vi "MAIN.vi"() -> ()   [LabVIEW 2015]
doc: "Use this template to create an application that executes repeatedly until you click the Stop button. This template polls the state of the Stop button and does not use events. Use the Top-Level Application template (not available in the Base package) to create a single-loop application with event handling."
uses:
  Lib_Bled112 toolkit/type_def/connection_status_bundle.ctl
  Lib_Bled112 toolkit/type_def/address_type.ctl
  Lib_Bled112 toolkit/type_def/message_type.ctl
  Lib_Bled112 toolkit/type_def/message_class.ctl
  <vilib>/Utility/miscctls.llb/LVPointTypeDef.ctl
  SUB_Load and Save Controls.llb/RWC_Actions.ctl
  <vilib>/Utility/miscctls.llb/LVRowAndColumnTypeDef.ctl
  <vilib>/event_ctls.llb/eventvkey.ctl
  <vilib>/Utility/sysdir.llb/System Directory Type.ctl
  <vilib>/Utility/NIReport.llb/image depth.ctl
  <vilib>/Analysis/baseanly.llb/Mean (DBL).vi
  Global 1.vi
  <vilib>/Utility/config.llb/Read Key (String).vi
  <vilib>/Utility/config.llb/Read Key (I32).vi
  Lib_Bled112 toolkit/ble_functions/ble_write_by_handle_uint8array.vi
  <vilib>/addons/_office/excel.llb/Excel Easy Table (str).vi
  <vilib>/Utility/config.llb/Write Key (String).vi
  <vilib>/Utility/config.llb/Write Key (U32).vi
  <vilib>/Utility/NIReport.llb/NI_report.lvclass
  <vilib>/Utility/config.llb/NI_LVConfig.lvlib
  <vilib>/Analysis/NI_AALBase.lvlib
  <vilib>/addons/_office/NI_ReportGenerationToolkit.lvlib
  <vilib>/Utility/NIReport.llb/NI_ReportGenerationCore.lvlib
  <vilib>/Utility/NIReport.llb/Excel/NI_Excel.lvclass
  <vilib>/Analysis/NI_AALPro.lvlib
panel:
  out "ms timer 3":u32=25058615
  in  "Interval(ms)":u16
  out "ms timer 2":u32=25058615
  out "Rx-ROM":bool=TRUE
  out "BLE Packet (mon)":u8[](array[numeric])
  out "Timer-ble log":u32
  out "log data1":bool=TRUE
  out "log ble buf":string
  out "Packet Detect":bool=TRUE
  out "Disconnected":bool=TRUE
  out "Rx OK":bool=TRUE
  out "Rx buf 1":string
  out "Rx Cnt":i32=3775
  out "Rx Packet Structure":T1={"Message Type (Response)"=128, "Payload length"=0, "Command Class (System)"=1, "Message ID"=0, "Connection handle"=0, "Attribute handle"=0, "Attribute type"=1, "Attribute value (data)"=[]} {"Attribute type" format="%02x" items=["read", "notify", "indicate", "read_by_type", "read_blob", "indicate_rsp_req"]; "Attribute value (data)" format="%02x"; "Attribute handle" format="%04x"; "Connection handle" format="%02x"; "Message ID" format="%02x"; "Message Type (Response)" format="%02x" items=["Command / Response"=0, "Event"=128]; "Command Class (System)" format="%02x" items=["System", "Persistent Store", "Attribute database", "Connection", "Attribute client", "Security Manager", "Generic Access Profile", "Hardware"]}
  out "Device Name":string
  out "Connection Status":T4={"MAC Address"="D9:2F:10:92:34:F2", "cnx handle"=0, "cnx flags"=5, "Address Type"=1, "Connection Interval (ms)"=15, "Timeout(ms)"=1000, "Latency"=0, "bonding handle"=255} {"Address Type" items=["Public", "Random"]}
  in  "Log no":string="1" caption="No."
  out "FTS OP status":T6="시험 시작"
  out "Test profile":string[][](array[string])=[["Init(1)-35lb", "35", "5000"], ["Init(2)-70lb", "70", "5000"], ["Load(1)-0lb", "0", "3000"], ["Load(2)-5lb", "5", "3000"], ["Load(3)-10lb", "10", "3000"], ["Load(4)-20lb", "20", "3000"], ["Load(5)-30lb", "30", "3000"], ["Load(6)-40lb", "40", "3000"]]
  out "log refnum":refnum<file> caption="참조 번호 복제"
  out "ms timer":u32=25058615
  out "Logging No.":u32
  in  "Data Logging":bool caption="Data Logging (Desktop folder)"
  out "RxD":string
  out "Graph timer 2":u32=25058662
  out "창크게":bool
  out "Comm err cnt 1":i32
  out "Graph timer 1":u32=25058662
  in  "Setting load":bool=TRUE
  out "ACT-Comm":bool
  in  "Comm con 1":bool
  in  "Port close 1":bool
  in  "Port open 1":bool
  in  "탭-Top":T7(tab)
  out "CDC Offet":T8 caption="CDC Offset data" {"Right Wing-C, C6/C0" format="%#.9f"; "Right Wing-B, C5/C0" format="%#.9f"; "Right Wing-A, C4/C0" format="%#.9f"; "Left Wing-C, C3/C0" format="%#.9f"; "Left Wing-B, C2/C0" format="%#.9f"; "Left Wing-A, C1/C0" format="%#.9f"}
  in  "Export graph 1":bool
  in  "Clear graph 1":bool
  out "CDC(PCAP02) Graph":waveform(dbl)[](graph)=[{"t0"=timestamp(3554680480.5032296 s since 1904-01-01), "dt"=0.10200000000000001, "Y"=[0.9929709434509277]}, {"t0"=timestamp(3554680480.5032296 s since 1904-01-01), "dt"=0.10200000000000001, "Y"=[0.9975447654724121]}, {"t0"=timestamp(3554680480.5032296 s since 1904-01-01), "dt"=0.10200000000000001, "Y"=[0.9987750053405762]}, {"t0"=timestamp(3554680480.5032296 s since 1904-01-01), "dt"=0.10200000000000001, "Y"=[1.0097055435180664]}, {"t0"=timestamp(3554680480.5032296 s since 1904-01-01), "dt"=0.10200000000000001, "Y"=[1.0132465362548828]}, {"t0"=timestamp(3554680480.5032296 s since 1904-01-01), "dt"=0.10200000000000001, "Y"=[1.0090084075927734]}]
  out "CDC data":T8 caption="CDC Monitoring data" {"Right Wing-C, C6/C0" format="%#.9f"; "Right Wing-B, C5/C0" format="%#.9f"; "Right Wing-A, C4/C0" format="%#.9f"; "Left Wing-C, C3/C0" format="%#.9f"; "Left Wing-B, C2/C0" format="%#.9f"; "Left Wing-A, C1/C0" format="%#.9f"}
  in  "Offset 1":bool
  out "IMU Offet":T9 caption="IMU Offset data" {"Accelerometer Z" format="%#.9f"; "Accelerometer Y" format="%#.9f"; "Accelerometer X" format="%#.9f"; "Gyroscope Z" format="%#.9f"; "Gyroscope Y" format="%#.9f"; "Gyroscope X" format="%#.9f"}
  out "IMU Graph":waveform(dbl)[](graph)=[{"t0"=timestamp(3554680480.5032296 s since 1904-01-01), "dt"=0.10200000000000001, "Y"=[3.465625]}, {"t0"=timestamp(3554680480.5032296 s since 1904-01-01), "dt"=0.10200000000000001, "Y"=[-2.45625]}, {"t0"=timestamp(3554680480.5032296 s since 1904-01-01), "dt"=0.10200000000000001, "Y"=[-1.45875]}, {"t0"=timestamp(3554680480.5032296 s since 1904-01-01), "dt"=0.10200000000000001, "Y"=[-0.014274]}, {"t0"=timestamp(3554680480.5032296 s since 1904-01-01), "dt"=0.10200000000000001, "Y"=[0.000305]}, {"t0"=timestamp(3554680480.5032296 s since 1904-01-01), "dt"=0.10200000000000001, "Y"=[1.025959]}]
  in  "Clear graph 2":bool
  in  "Export graph2":bool
  out "IMU data":T9 caption="IMU Monitoring data" {"Accelerometer Z" format="%#.9f"; "Accelerometer Y" format="%#.9f"; "Accelerometer X" format="%#.9f"; "Gyroscope Z" format="%#.9f"; "Gyroscope Y" format="%#.9f"; "Gyroscope X" format="%#.9f"}
  in  "Offset 2":bool
  out "Full ROM data":bool
  in  "Flash Map":enum32{"Data Map", "Raw Data"}(tab)
  out "Rx ROM-log":string
  out "ROM Data":T10(array[cluster]) {"Index" format="%02x"; "ROM Data" format="%02x"}
  out "Bat(raw)":u16 format="%04x"
  in  "Load(lb)":dbl=10.0 min=0.0 max=150.0 step=0.1
  in  "Test name":string="Noname"
  out "Load vs Ratio Graph":cluster{dbl[], dbl[]}[](graph)
  in  "Mark10 Gauge (lb)":dbl format="%.2f"
  out "Test Status":string
  out "Test Data table":string[][](table)=[["-", "-", "-", "-", "-", "-", "-", "-", "-", "-"], ["-", "-", "-", "-", "-", "-", "-", "-", "-", "-"], ["-", "-", "-", "-", "-", "-", "-", "-", "-", "-"], ["-", "-", "-", "-", "-", "-", "-", "-", "-", "-"], ["-", "-", "-", "-", "-", "-", "-", "-", "-", "-"], ["-", "-", "-", "-", "-", "-", "-", "-", "-", "-"], ["-", "-", "-", "-", "-", "-", "-", "-", "-", "-"], ["-", "-", "-", "-", "-", "-", "-", "-", "-", "-"], ["-", "-", "-", "-", "-", "-", "-", "-", "-", "-"]]
  in  "Test Start":bool
  in  "Port-FTS":refnum<visa-resource-name>="COM5" caption="FTS \nCOM port"
  in  "FTS Testing":bool
  out "FTS comm.":bool
  in  "Force Set":bool
  out "Rx-mon":bool=TRUE
  out "Comm con status 1":bool caption="Status"
  out "*Board ID1":string="None...." caption="S/N"
  in  "Port-set 1":refnum<visa-resource-name>="COM4" caption="COM port"
  out "Port-act 1":refnum<visa-resource-name>="COM4"
  in  "stop":bool=TRUE
  out "Data trx(led)":bool
  in  "Setting load(led)":bool
  out "status string":string="Ready (available after the communication connection)"
  # "GEN4 2nd PP - GUI Program"
  # "Ver. 161109A"
  # "Comm. Connection"
  # "115200bps"
  # "Gyroscope X"
  # "Gyroscope Y"
  # "Gyro. (dps)"
  # "Gyroscope Z"
  # "Accelerometer X"
  # "Accelerometer Y"
  # "Acc. (g)"
  # "Accelerometer Z"
  # "Reserved"
  # "ESM301: 115200bps\nMARK10: 9600bps"
  # "<Response test>"
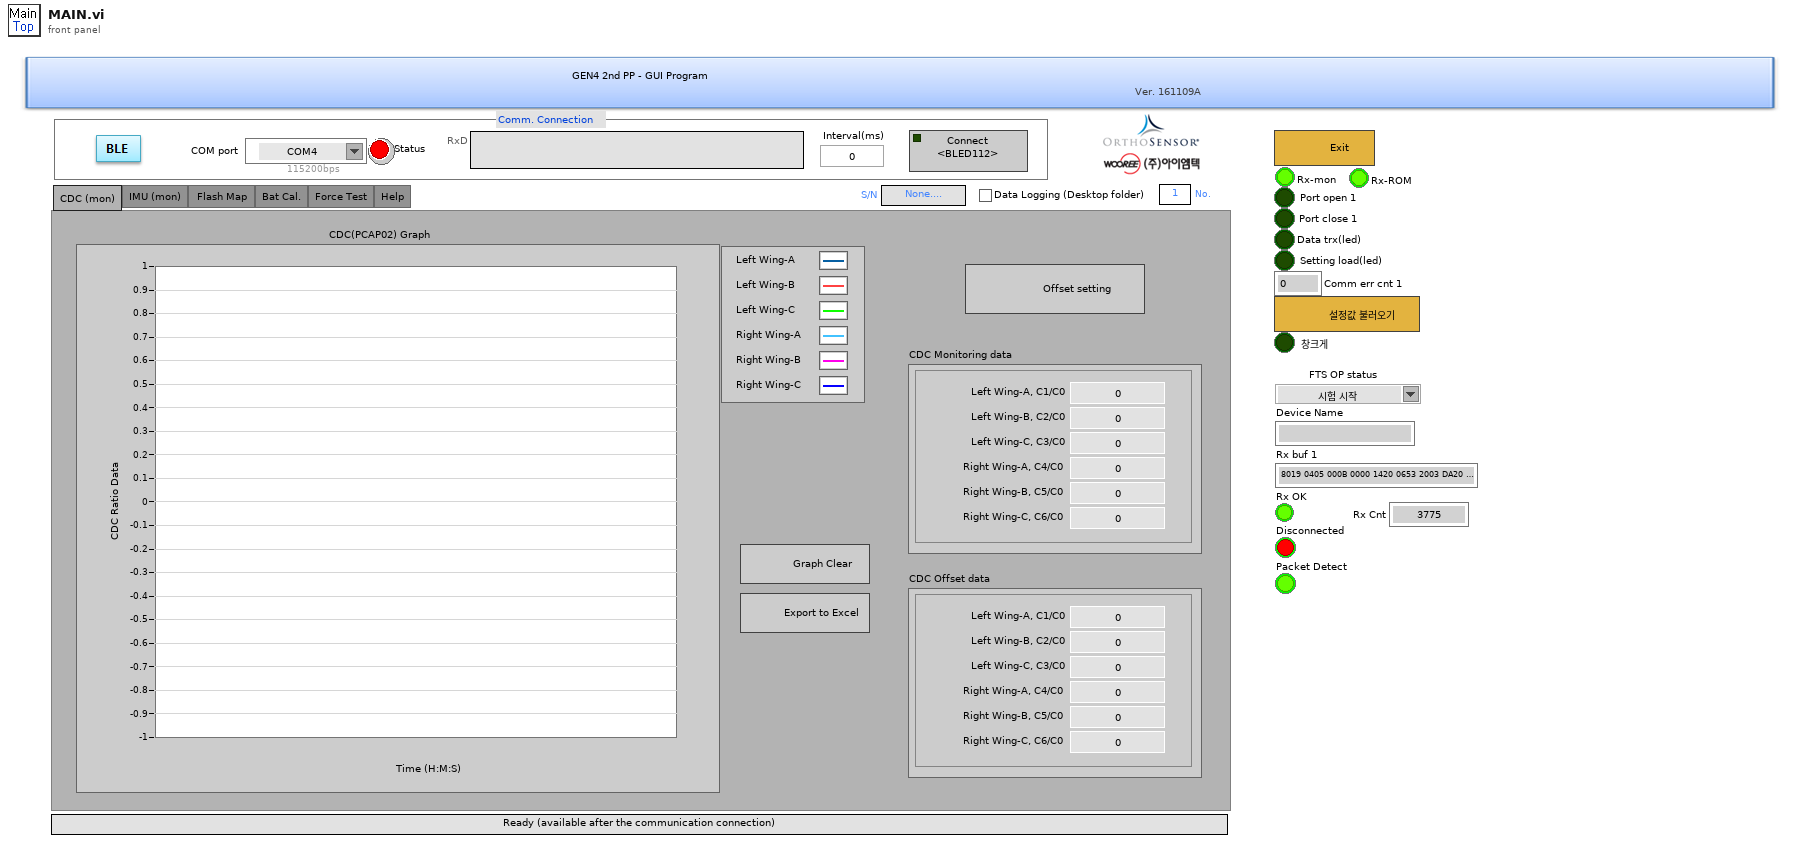
[diagram p1: front panel]
types:
  T1 = typedef "컨트롤-BLED Rx (EVENT-Attribute Client).ctl" = cluster{"Message Type (Response)":T2, "Payload length":u8, "Command Class (System)":T3, "Message ID":u8, "Connection handle":u8, "Attribute handle":u16, "Attribute type":T3, "Attribute value (data)":u8[]}
  T2 = typedef "message_type.ctl" = u8
  T3 = typedef "message_class.ctl" = u8
  T4 = typedef "connection_status_bundle.ctl" = cluster{"MAC Address":string, "cnx handle":u8, "cnx flags":u8, "Address Type":T5, "Connection Interval (ms)":u16, "Timeout(ms)":u16, "Latency":u16, "bonding handle":u8}
  T5 = typedef "address_type.ctl" = u8
  T6 = typedef "컨트롤-동작시험상태 FTS.ctl" = string
  T7 = enum32{"CDC (mon)", "IMU (mon)", "Flash Map ", "Bat Cal.", "Force Test", "Help"}
  T8 = typedef "컨트롤-CDC data.ctl" = cluster{"Left Wing-A, C1/C0":dbl, "Left Wing-B, C2/C0":dbl, "Left Wing-C, C3/C0":dbl, "Right Wing-A, C4/C0":dbl, "Right Wing-B, C5/C0":dbl, "Right Wing-C, C6/C0":dbl}
  T9 = typedef "컨트롤-IMU data.ctl" = cluster{"Gyroscope X":dbl, "Gyroscope Y":dbl, "Gyroscope Z":dbl, "Accelerometer X":dbl, "Accelerometer Y":dbl, "Accelerometer Z":dbl}
  T10 = cluster{"RxOK":bool, "ROM Data":u8[], "Index":u8}[]
  T11 = typedef "RWC_Actions.ctl" = enum16{"Read", "Write", "Read and Create"}
  T12 = enum16{"Always On", "Always Off", "Off While Running"}
  T13 = typedef "LVPointTypeDef.ctl" = cluster{"Horizontal":i16, "Vertical":i16}
  T14 = cluster{"RxOK":bool, "ROM Data":u8[], "Index":u8}
  T15 = typedef "LVRowAndColumnTypeDef.ctl" = cluster{"Row":i32, "Column":i32}
  T16 = typedef "컨트롤-동작상태 FTS.ctl" = string
  T17 = typedef "eventvkey.ctl" = enum16{"ASCII", "Enter", "Return", "Shift", "Ctrl", "Alt", "Cmd", "Opt", "Caps", "NumLock", "Clear", "Break", "Up", "Down", "Left", "Right", "Insert", "Delete", "Home", "End", "PageUp", "PageDown", "Escape", "Help", "Pause", "ScrollLock", "F1", "F2", "F3", "F4", "F5", "F6", "F7", "F8", "F9", "F10", "F11", "F12", "F13", "F14", "F15", "F16", "F17", "F18", "F19", "F20", "F21", "F22", "F23", "F24", "Play", "VolumeUp", "VolumeDown", "Mute", "Two Byte Char"}
  T18 = cluster{"position (Excel)":cluster{"row":i32, "column":i32}, "name (Excel)":string, "bookmark (Word)":string}
  T19 = enum16{"Standard Report", "HTML", "Word", "Excel"}
  T20 = enum16{"maximized", "minimized", "normal", "no change"}
  T21 = typedef "컨트롤-설정값 선택.ctl" = string
  T22 = enum16{"open", "replace", "create", "open or create", "replace or create", "replace or create with confirmation"}
  T23 = typedef "NI_LVConfig.lvlib/Config Data RefNum.ctl" = refnum<k1>
  T24 = typedef "System Directory Type.ctl" = i32
  T25 = typedef "NI_ReportGenerationCore.lvlib/image depth.ctl" = u16
  T26 = typedef "LVRectTypeDef.ctl" = cluster{"Left":i16, "Top":i16, "Right":i16, "Bottom":i16}
  T27 = typedef "컨트롤-BLED Rx (EVENT-Connection status).ctl" = cluster{"Message Type (Response)":T2, "Payload length":u8, "Command Class (System)":T3, "Message ID":u8, "Connection handle":u8, "flags":u8, "Bluetooth address":u8[], "address type":T3, "conn_interval(ms)":dbl, "timeout(ms)":dbl, "latency":u16, "bonding(0xFF)":u8}
  T28 = typedef "컨트롤-BLED Rx (EVENT-Disconnected).ctl" = cluster{"Message Type (Response)":T2, "Payload length":u8, "Command Class (Connection)":T3, "Message ID":u8, "connection":u8, "reason":u16}
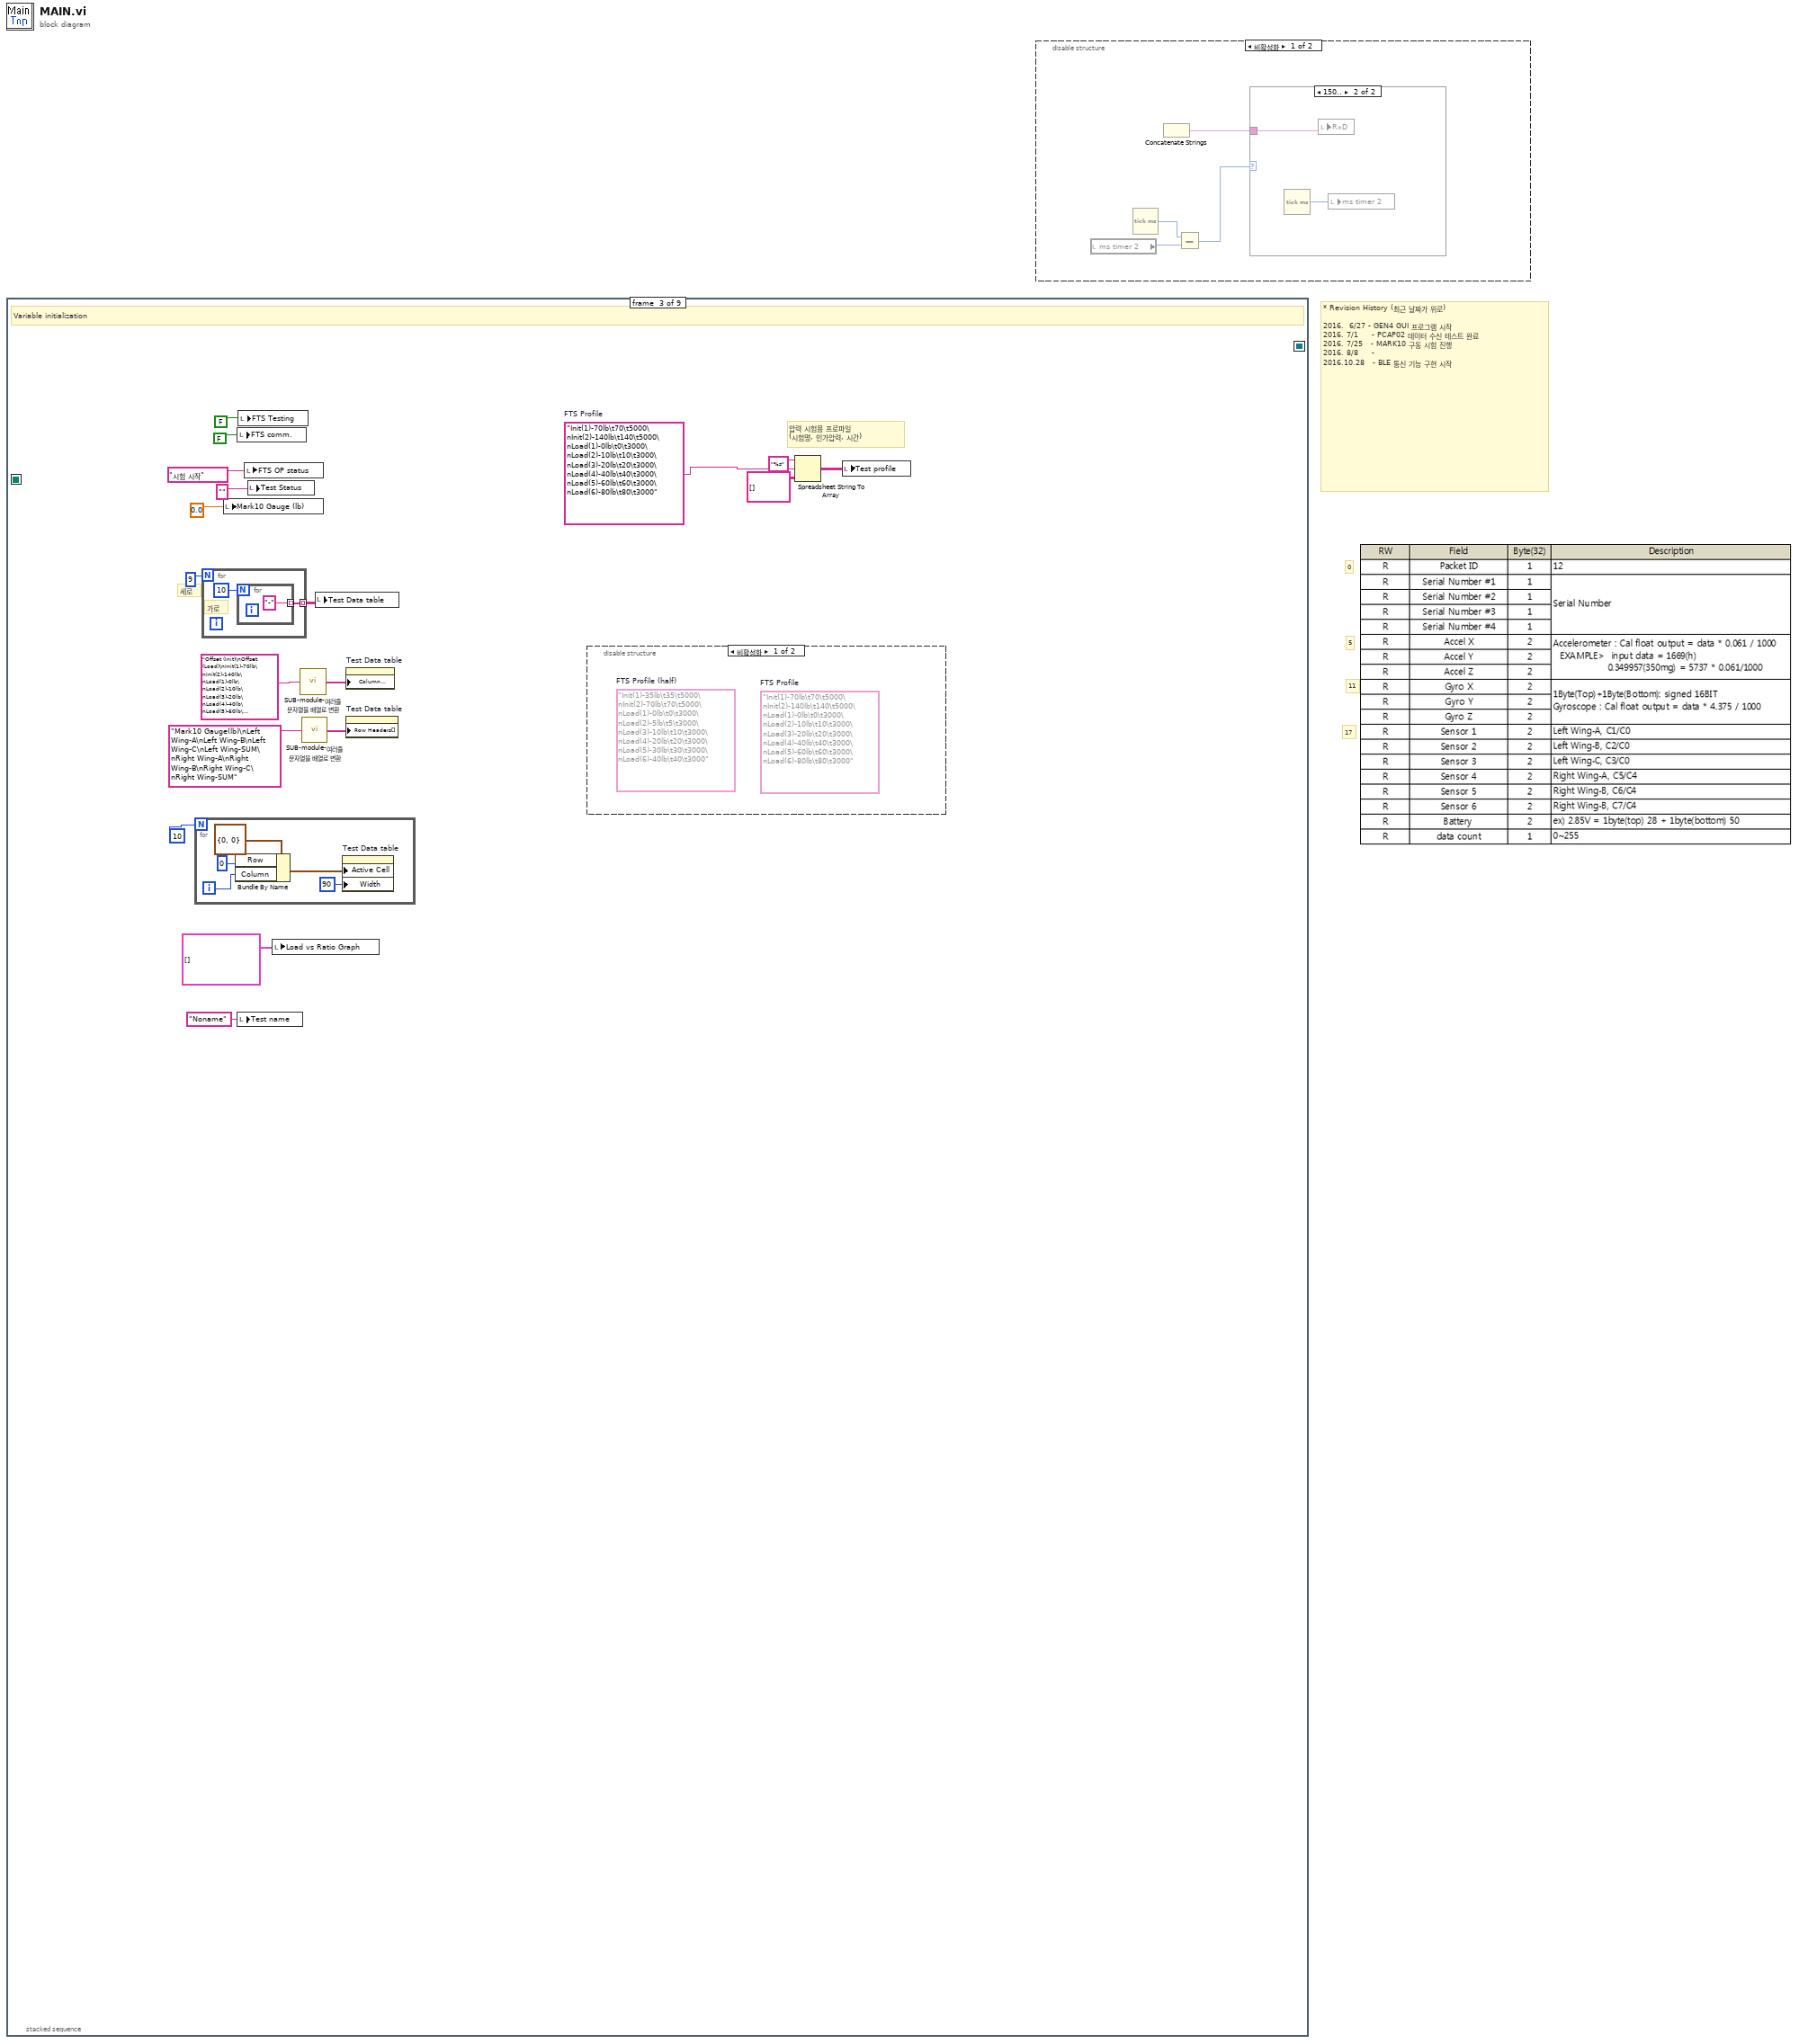
[diagram p0: block diagram]
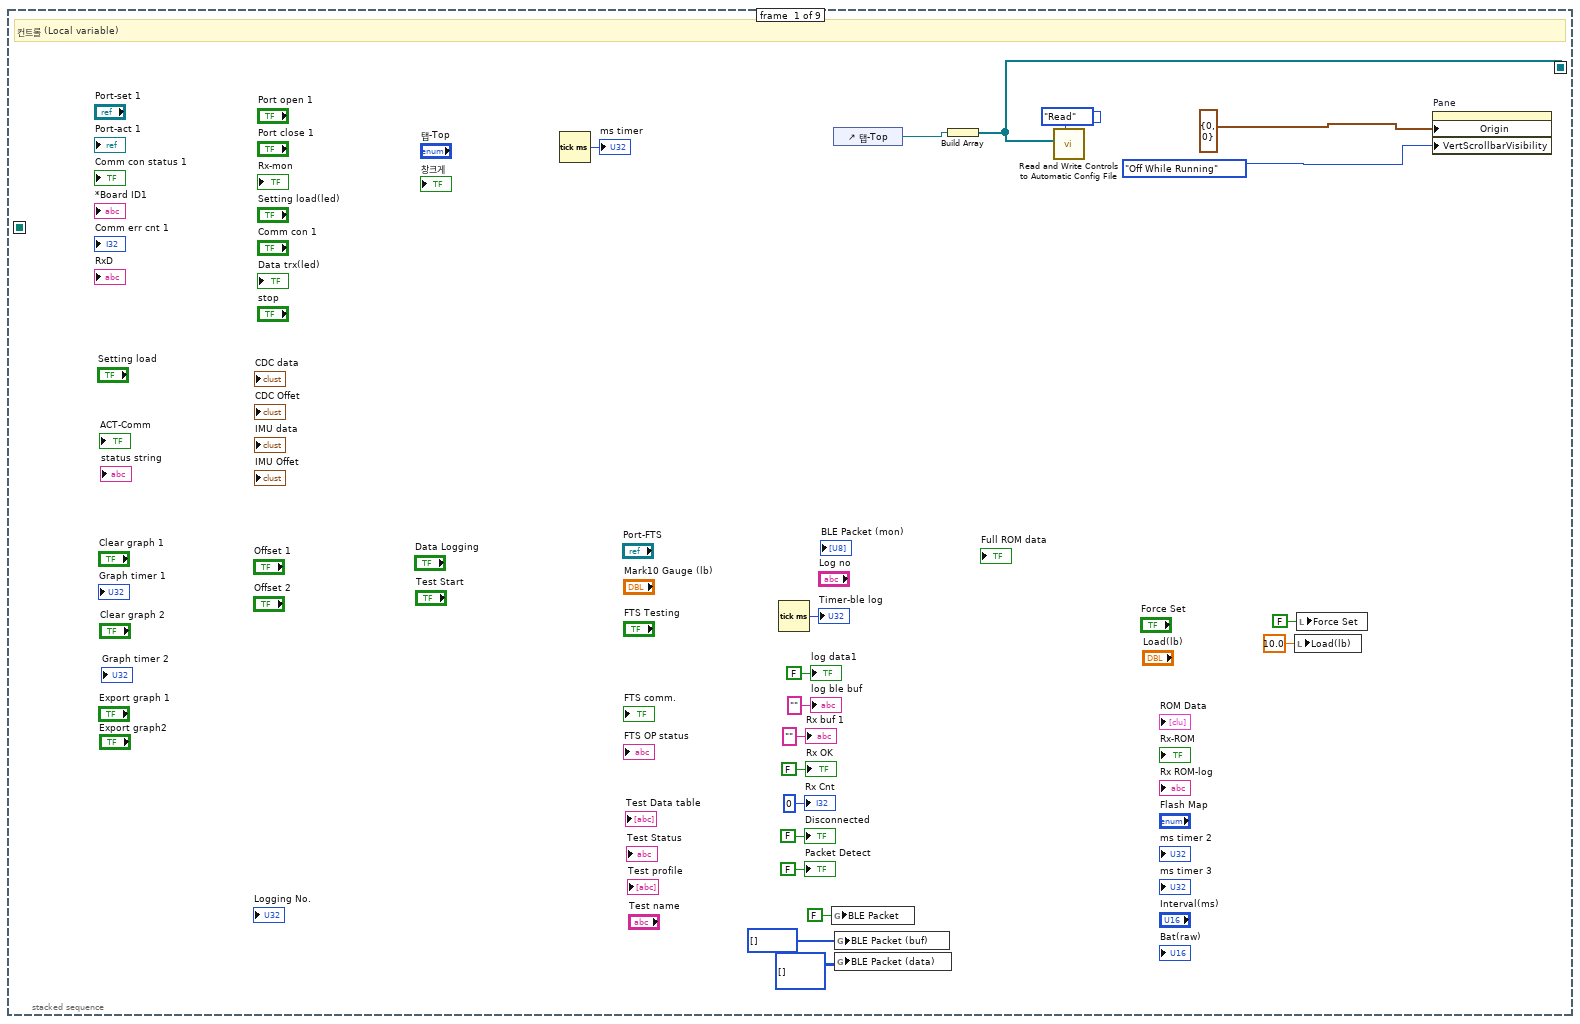
[diagram p4: hidden frame]
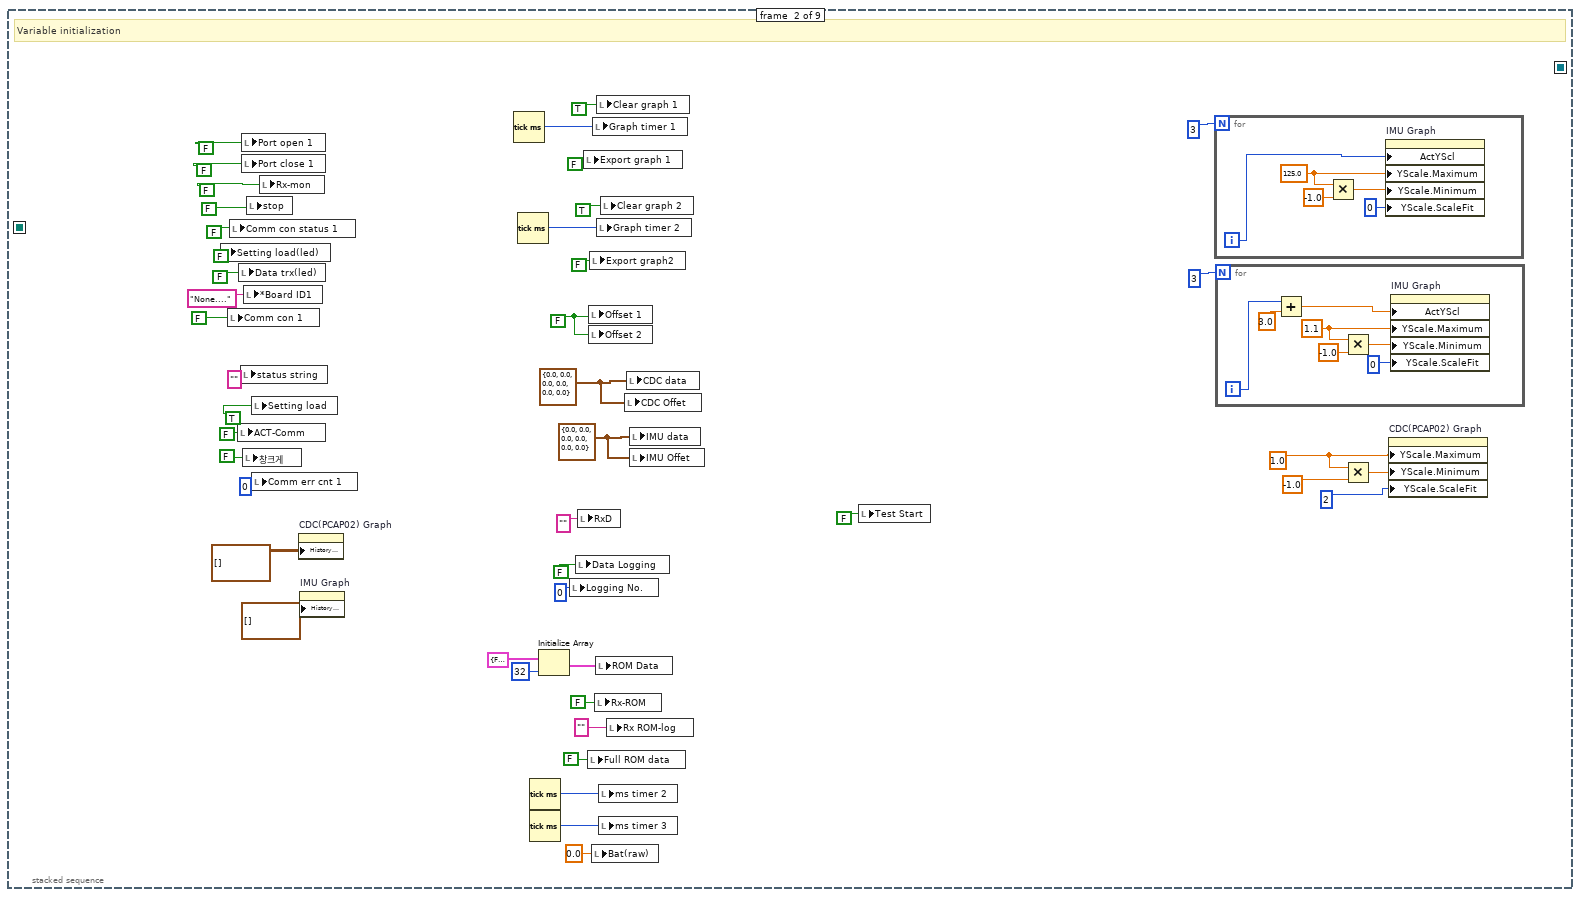
[diagram p5: hidden frame]
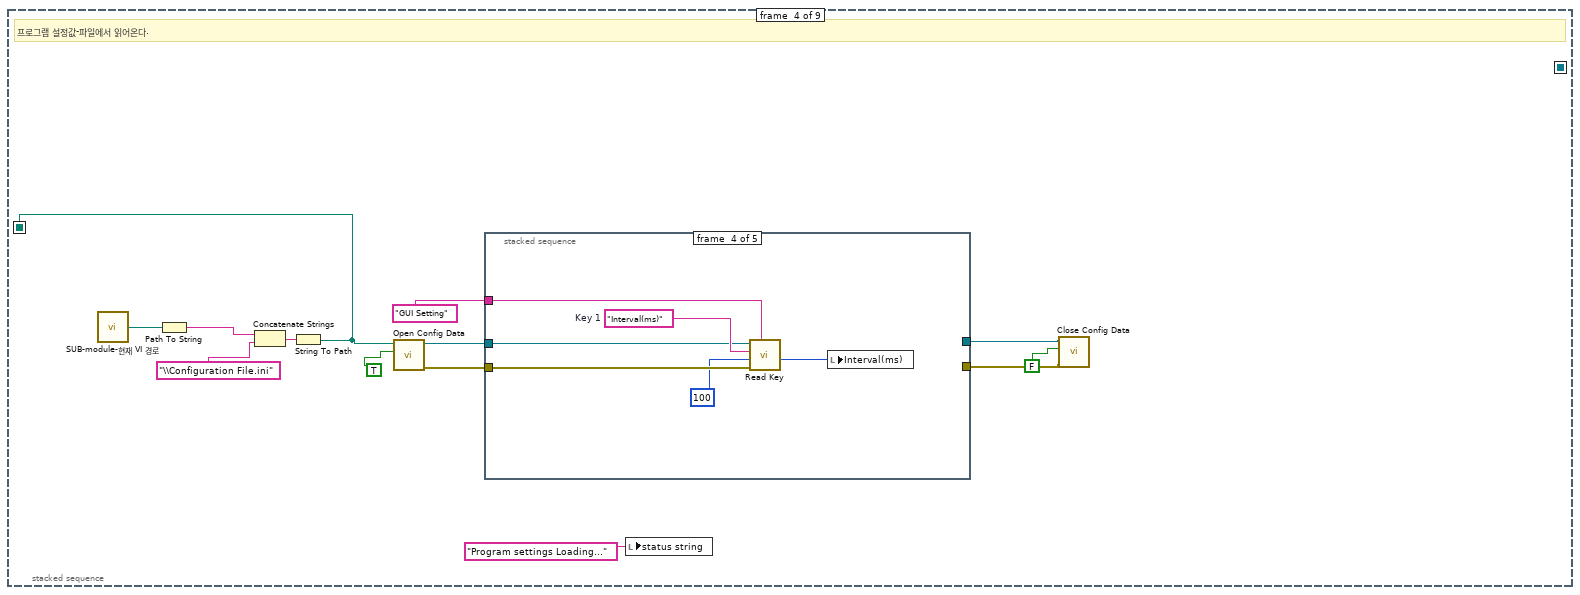
[diagram p7: hidden frame]
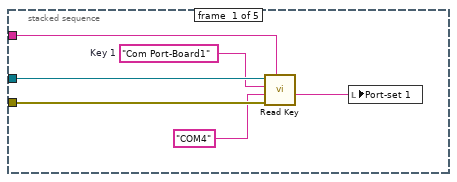
[diagram p8: hidden frame]
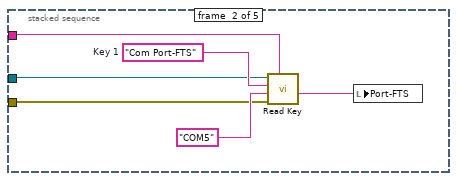
[diagram p9: hidden frame]
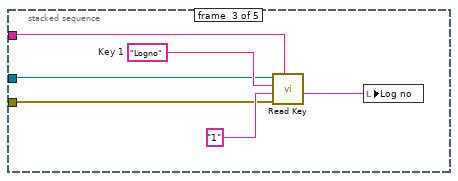
[diagram p10: hidden frame]
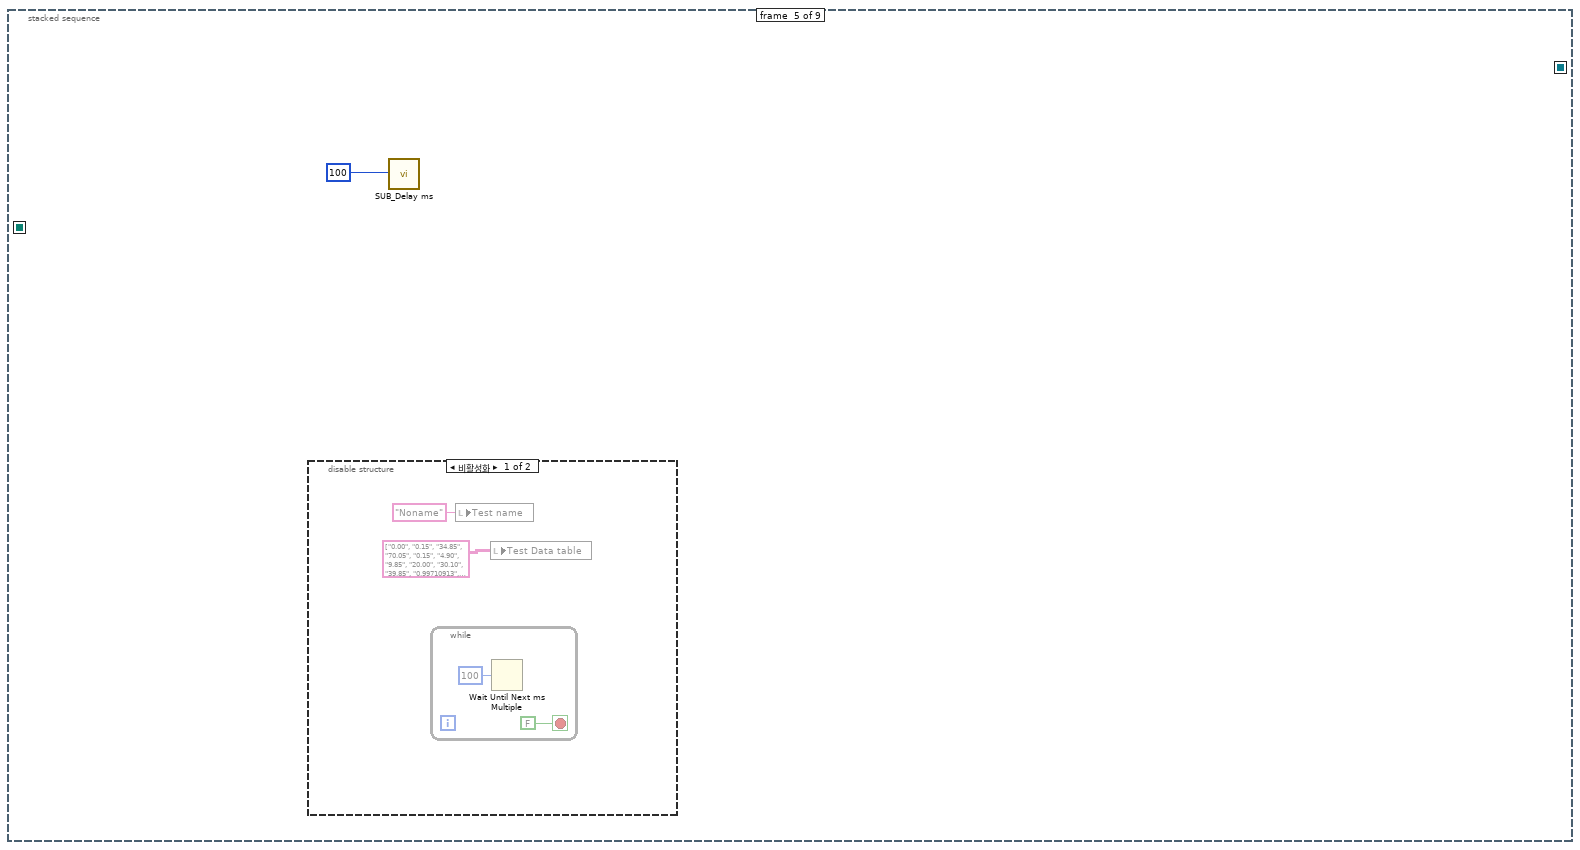
[diagram p12: hidden frame]
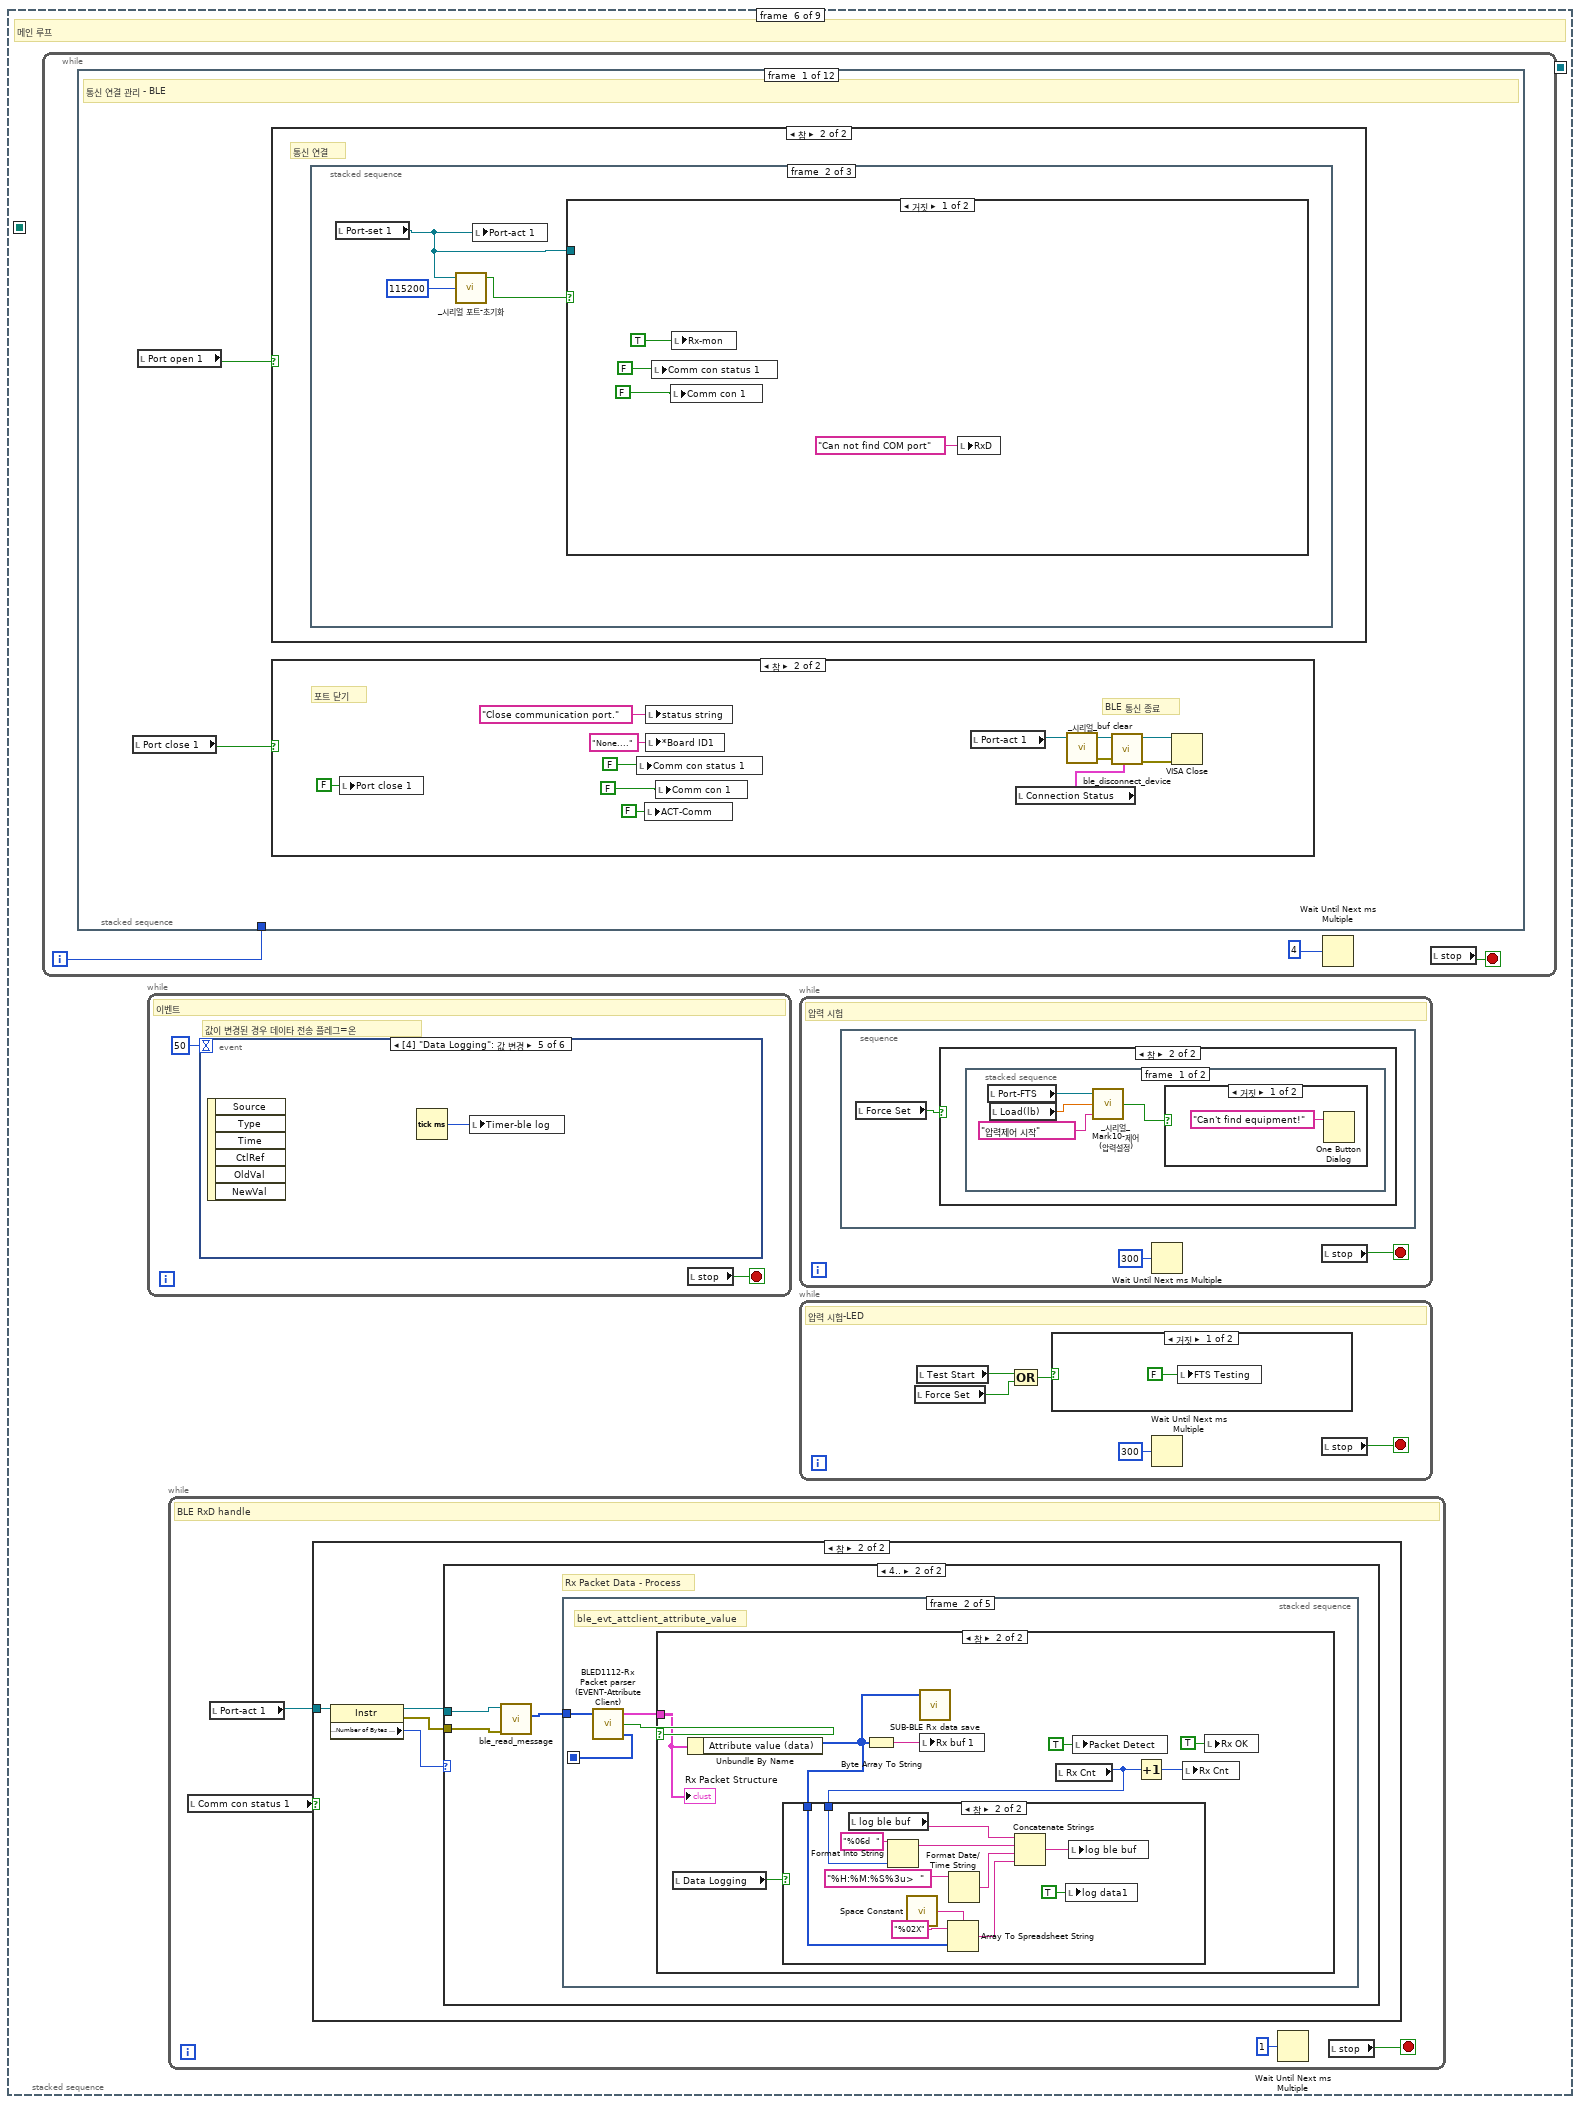
[diagram p14: hidden frame]
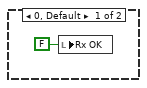
[diagram p16: hidden frame]
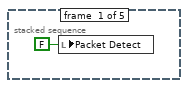
[diagram p17: hidden frame]
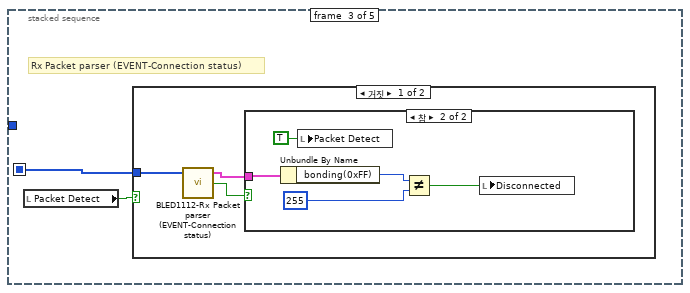
[diagram p20: hidden frame]
diagram:
  # "17"
  # "11"
  # "5"
  # "0"
  # "* Revision History (최근 날짜가 위로)\n\n2016.  6/27 - GEN4 GUI 프로그램 시작\n2016. 7/1     - PCAP02 데이터 수신 테스트 완료\n2016. 7/25   - MARK10 구동 시험 진행\n2016. 8/8     -  \n2016.10.28   - BLE 통신 기능 구현 시작"
  n1 = stacked-sequence {
    seq-local: [_ _ _ w106 _ _ _ _ _] -> [_ _ _ _ _ _ _ w1111 _]
    seq-local: [w17 _ _ _ _ _ _ _ _] -> [_ _ _ _ _ _ _ w1107 _]
    frame #0 {
      # "컨트롤 (Local variable)"
      n2 = Tick Count (ms)() -> (millisecond timer value=→"ms timer":u32)
      n3 = Tick Count (ms)() -> (millisecond timer value=→"Timer-ble log":u32)
      n4 = global write "Global 1.vi" "BLE Packet"(FALSE ("BLE Packet")) -> ()
      n5 = control-ref of="탭-Top"() -> (w15:refnum<vi>)
      n6 = global write "Global 1.vi" "BLE Packet (buf)"(u8[] [] ("BLE Packet (buf)")) -> ()
      n7 = global write "Global 1.vi" "BLE Packet (data)"(u8[][] [] ("BLE Packet (data)")) -> ()
      n8 = Build Array(w15) -> (w17:refnum<vi>[])
      n9 = call "Read and Write Controls to Automatic Config File.vi"("Action"=RWC_Actions."Read", "Control References"=w17) -> ()  [unwired: 9 in, 1 out]
      n10 = local write "Load(lb)"(10.0 ("Load(lb)")) -> ()
      n11 = local write "Force Set"(FALSE ("Force Set")) -> ()
      n12 = property on="Pane" class="Pane"("Origin"=T13 {"Horizontal"=0, "Vertical"=0} ("원점"), "VertScrollbarVisibility"=T12."Off While Running" ("수직 스크롤 막대 보이기")) -> ()  [unwired: 2 in, 2 out]
      "Rx Cnt" <- 0 ("Rx Cnt")
      "Rx buf 1" <- "" ("Rx 문자열 1")
      "Rx OK" <- FALSE ("Rx OK")
      "Disconnected" <- FALSE ("Disconnected")
      "Packet Detect" <- FALSE ("Packet Detect")
      "log ble buf" <- "" ("log ble buf")
      "log data1" <- FALSE ("log data1")
    }
    frame #1 {
      w34 = 1.0 ("Y 스케일.범위:최대값")
      w40 = T9 {"Gyroscope X"=0.0, "Gyroscope Y"=0.0, "Gyroscope Z"=0.0, "Accelerometer X"=0.0, "Accelerometer Y"=0.0, "Accelerometer Z"=0.0} ("IMU data")
      w41 = T8 {"Left Wing-A, C1/C0"=0.0, "Left Wing-B, C2/C0"=0.0, "Left Wing-C, C3/C0"=0.0, "Right Wing-A, C4/C0"=0.0, "Right Wing-B, C5/C0"=0.0, "Right Wing-C, C6/C0"=0.0} ("CDC data")
      w42 = FALSE ("Offset 1")
      # "Variable initialization"
      n13 = local write "Setting load(led)"(FALSE ("Power On Flag")) -> ()
      n14 = local write "Comm con 1"(FALSE ("포트 연결")) -> ()
      n15 = local write "Comm con status 1"(FALSE ("Connected")) -> ()
      n16 = local write "ACT-Comm"(FALSE ("ACT-RS422")) -> ()
      n17 = local write "Data trx(led)"(FALSE ("Rx")) -> ()
      n18 = local write "status string"("" ("status string")) -> ()
      n19 = local write "Port open 1"(FALSE) -> ()
      n20 = local write "Port close 1"(FALSE) -> ()
      n21 = local write "창크게"(FALSE ("창크게")) -> ()
      n22 = local write "*Board ID1"("None...." ("*Board ID")) -> ()
      n23 = local write "stop"(FALSE ("stop")) -> ()
      n24 = local write "Setting load"(TRUE ("설정값 불러오기")) -> ()
      n25 = local write "Comm err cnt 1"(0 ("통신에러카운트")) -> ()
      n26 = local write "Rx-mon"(FALSE) -> ()
      n27 = property on="CDC(PCAP02) Graph" class="WFChart (엄격한)"("History Data"=waveform(dbl)[][] [] ("히스토리 데이터")) -> ()  [unwired: 2 in, 2 out]
      n28 = property on="IMU Graph" class="WFChart (엄격한)"("History Data"=waveform(dbl)[][] [] ("히스토리 데이터")) -> ()  [unwired: 2 in, 2 out]
      n29 = Tick Count (ms)() -> (millisecond timer value=w51:u32)
      n30 = Tick Count (ms)() -> (millisecond timer value=w44:u32)
      n31 = Tick Count (ms)() -> (millisecond timer value=w26:u32)
      n32 = Tick Count (ms)() -> (millisecond timer value=w27:u32)
      n33 = Initialize Array(T14 {"RxOK"=FALSE, "ROM Data"=[], "Index"=0} ("클러스터"), 32 ("차원 크기")) -> (w22:T10)
      n34 = local write "Logging No."(u32 0 ("Logging No.")) -> ()
      n35 = local write "Data Logging"(FALSE ("Data Logging")) -> ()
      n36 = local write "RxD"("" ("RxD")) -> ()
      n37 = local write "Export graph 1"(FALSE ("그래프 반출")) -> ()
      n38 = local write "Full ROM data"(FALSE ("Full ROM data")) -> ()
      n39 = local write "Offset 1"(w42) -> ()
      n40 = local write "Offset 2"(w42) -> ()
      n41 = local write "Export graph2"(FALSE ("그래프 반출")) -> ()
      n42 = local write "Bat(raw)"(0.0 ("Bat(raw)")) -> ()
      n43 = local write "Graph timer 1"(w51) -> ()
      n44 = local write "Rx-ROM"(FALSE ("Rx-ROM")) -> ()
      n45 = local write "ROM Data"(w22) -> ()
      n46 = local write "Clear graph 1"(TRUE ("그래프 지우기")) -> ()
      n47 = local write "Graph timer 2"(w44) -> ()
      n48 = local write "ms timer 2"(w26) -> ()
      n49 = local write "ms timer 3"(w27) -> ()
      n50 = local write "Clear graph 2"(TRUE ("그래프 지우기")) -> ()
      n51 = local write "Rx ROM-log"("" ("문자열-Rx ROM")) -> ()
      n52 = local write "CDC Offet"(w41) -> ()
      n53 = local write "CDC data"(w41) -> ()
      n54 = local write "IMU data"(w40) -> ()
      n55 = local write "IMU Offet"(w40) -> ()
      n56 = local write "Test Start"(FALSE ("Test Start")) -> ()
      n57 = for {
        N: 3 -> [_]
        i -> [w72]
        w73 = 125.0 ("Y 스케일.범위:최대값")
        n58 = Multiply(x=w73, y=-1.0 ("Y 스케일.범위:최대값")) -> (x*y=w75:dbl)
        n59 = property on="IMU Graph" class="WFChart (엄격한)"("ActYScl"=w72, "YScale.Maximum"=w73, "YScale.Minimum"=w75, "YScale.ScaleFit"=u8 0 ("Y 스케일.스케일 맞춤")) -> ()  [unwired: 2 in, 2 out]
      }
      n60 = for {
        N: 3 -> [_]
        i -> [w67]
        w68 = 1.1 ("Y 스케일.범위:최대값")
        n61 = Add(x=w67, y=3.0 ("Y 스케일.범위:최대값")) -> (x+y=w65:dbl)
        n62 = Multiply(x=w68, y=-1.0 ("Y 스케일.범위:최대값")) -> (x*y=w70:dbl)
        n63 = property on="IMU Graph" class="WFChart (엄격한)"("ActYScl"=w65, "YScale.Maximum"=w68, "YScale.Minimum"=w70, "YScale.ScaleFit"=u8 0 ("Y 스케일.스케일 맞춤")) -> ()  [unwired: 2 in, 2 out]
      }
      n64 = Multiply(x=w34, y=-1.0 ("Y 스케일.범위:최대값")) -> (x*y=w33:dbl)
      n65 = property on="CDC(PCAP02) Graph" class="WFChart (엄격한)"("YScale.Maximum"=w34, "YScale.Minimum"=w33, "YScale.ScaleFit"=u8 2 ("Y 스케일.스케일 맞춤")) -> ()  [unwired: 2 in, 2 out]
    }
    frame #2 {
      w76 = "Init(1)-70lb\t70\t5000\nInit(2)-140lb\t140\t5000\nLoad(1)-0lb\t0\t3000\nLoad(2)-10lb\t10\t3000\nLoad(3)-20lb\t20\t3000\nLoad(4)-40lb\t40\t3000\nLoad(5)-60lb\t60\t3000\nLoad(6)-80lb\t80\t3000"  # FTS Profile
      # "압력 시험용 프로파일\n(시험명, 인가압력, 시간)"
      # "세로"
      # "Variable initialization"
      n66 = for {
        N: 10 -> [_]
        i -> [w98]
        n67 = Bundle By Name(cluster=T15 {"Row"=0, "Column"=0} ("활성 셀:활성 셀"), "Row"=0, "Column"=w98) -> (w100:T15)
        n68 = property on="Test Data table" class="Tbl (엄격한)"("Active Cell"=w100, "Width"=u32 90 ("활성 셀:셀 크기:폭")) -> ()  [unwired: 2 in, 2 out]
      }
      n69 = for {
        N: 9 -> [_]
        tunnel: [w94] -> w84 mode=indexing
        # "가로"
        n70 = for {
          N: 10 -> [_]
          tunnel: ["-"] -> w94 mode=indexing
        }
      }
      n71 = local write "Mark10 Gauge (lb)"(0.0 ("Mark10 Gauge")) -> ()
      n72 = local write "FTS comm."(FALSE ("FTS 수신 정상")) -> ()
      n73 = local write "Test name"("Noname" ("Test name")) -> ()
      n74 = local write "FTS Testing"(FALSE ("FTS 시험 진행")) -> ()
      n75 = local write "FTS OP status"(T6 "시험 시작" ("FTS 동작시험 상태")) -> ()
      n76 = local write "Test Status"("" ("Force Test Status")) -> ()
      n77 = local write "Load vs Ratio Graph"(cluster{dbl[], dbl[]}[] [] ("Load vs Ratio Graph")) -> ()
      n78 = call "SUB-module-여러줄 문자열을 배열로 변환.vi"("문자열"="Offset (Init)\nOffset (Load)\nInit(1)-70lb\nInit(2)-140lb\nLoad(1)-0lb\nLoad(2)-10lb\nLoad(3)-20lb\nLoad(4)-40lb\nLoad(5)-60lb\nLoad(6)-80lb") -> ("배열"=w81:string[])
      n79 = call "SUB-module-여러줄 문자열을 배열로 변환.vi"("문자열"="Mark10 Gauge(lb)\nLeft Wing-A\nLeft Wing-B\nLeft Wing-C\nLeft Wing-SUM\nRight Wing-A\nRight Wing-B\nRight Wing-C\nRight Wing-SUM") -> ("배열"=w79:string[])
      n80 = local write "Test Data table"(w84) -> ()
      n81 = property on="Test Data table" class="Tbl (엄격한)"("Column Headers[]"=w81) -> ()  [unwired: 2 in, 2 out]
      n82 = property on="Test Data table" class="Tbl (엄격한)"("Row Headers[]"=w79) -> ()  [unwired: 2 in, 2 out]
      n83 = disable-structure shown="비활성화" {
        frame Disabled {
          (unwired) "Init(1)-35lb\t35\t5000\nInit(2)-70lb\t70\t5000\nLoad(1)-0lb\t0\t3000\nLoad(2)-5lb\t5\t3000\nLoad(3)-10lb\t10\t3000\nLoad(4)-20lb\t20\t3000\nLoad(5)-30lb\t30\t3000\nLoad(6)-40lb\t40\t3000"  # FTS Profile (half)
          (unwired) "Init(1)-70lb\t70\t5000\nInit(2)-140lb\t140\t5000\nLoad(1)-0lb\t0\t3000\nLoad(2)-10lb\t10\t3000\nLoad(3)-20lb\t20\t3000\nLoad(4)-40lb\t40\t3000\nLoad(5)-60lb\t60\t3000\nLoad(6)-80lb\t80\t3000"  # FTS Profile
        }
        frame Enabled {
        }
      }
      n84 = Spreadsheet String To Array(format string="%s" ("포맷 문자열"), spreadsheet string=w76, array type (2D Dbl)=string[][] [] ("배열 타입(2D Dbl)")) -> (array=w88:string[][])  [unwired: 1 in]
      n85 = local write "Test profile"(w88) -> ()
    }
    frame #3 {
      # "프로그램 설정값-파일에서 읽어온다."
      n86 = call "SUB-module-현재 VI 경로.vi"() -> ("현재 VI 경로"=w107:path)
      n87 = Path To String(path=w107) -> (string=w109:string)
      n88 = Concatenate Strings(w109, "\\Configuration File.ini") -> (w108:string)
      n89 = String To Path(string=w108) -> (path=w106:path)
      n90 = call <vilib>:"Open Config Data.vi"("create file if necessary (T)"=TRUE, "configuration file path"=w106) -> ("error out"=w113:errorcluster, "refnum"=w112:T23)  [unwired: 7 in, 1 out]
      n91 = stacked-sequence {
        tunnel: w112 -> [w120 w122 w128 w135 w140]
        tunnel: w113 -> [w119 w121 w127 w134 w139]
        tunnel: "GUI Setting" ("section") -> [w118 w123 w129 w136 _]
        tunnel: [_ _ _ _ w140] -> w104
        tunnel: [_ _ _ _ w139] -> w103
        frame #0 {
          w117 = "Com Port-Board1"  # Key 1
          n92 = call-poly <vilib>:"Read Key.vi"("section"=w118, "error in (no error)"=w119, "default value"="COM4" ("output string"), "key"=w117, "refnum"=w120) -> ("value"=w116:string)  [unwired: 3 in, 3 out]
          n93 = local write "Port-set 1"(w116) -> ()
        }
        frame #1 {
          w126 = "Com Port-FTS"  # Key 1
          n94 = call-poly <vilib>:"Read Key.vi"("section"=w123, "error in (no error)"=w121, "default value"="COM5" ("output string"), "key"=w126, "refnum"=w122) -> ("value"=w125:string)  [unwired: 3 in, 3 out]
          n95 = local write "Port-FTS"(w125) -> ()
        }
        frame #2 {
          w132 = "Logno"  # Key 1
          n96 = call-poly <vilib>:"Read Key.vi"("section"=w129, "error in (no error)"=w127, "default value"="1" ("output string"), "key"=w132, "refnum"=w128) -> ("value"=w131:string)  [unwired: 3 in, 3 out]
          n97 = local write "Log no"(w131) -> ()
        }
        frame #3 {
          w138 = "Interval(ms)"  # Key 1
          n98 = call-poly <vilib>:"Read Key.vi"("section"=w136, "error in (no error)"=w134, "default value"=100, "key"=w138, "refnum"=w135) -> ("value"=w137:i32)  [unwired: 3 in, 3 out]
          n99 = local write "Interval(ms)"(w137) -> ()
        }
        frame #4 {
        }
      }
      n100 = local write "status string"("Program settings Loading..." ("status string")) -> ()
      n101 = call <vilib>:"Close Config Data.vi"("error in (no error)"=w103, "write file if changed (T)"=FALSE ("write configuration file? (T)"), "refnum"=w104) -> ()  [unwired: 9 out]
    }
    frame #4 {
      n102 = disable-structure shown="비활성화" {
        frame Disabled {
          n103 = while {
            stop <- FALSE stop-if-true
            n104 = Wait Until Next ms Multiple(millisecond multiple=u32 100 ("ms 배수")) -> ()  [unwired: 1 out]
          }
          n105 = local write "Test name"("Noname" ("Test name")) -> ()
          n106 = local write "Test Data table"(string[][] [["0.00", "0.15", "34.85", "70.05", "0.15", "4.90", "9.85", "20.00", "30.10", "39.85"], ["0.99710913", "0.99710572", "0.00000334", "0.00000057", "0.00000226", "-0.00000107", "-0.00000546", "-0.00000098", "-0.00000517", "-0.00001023"], ["0.99966111", "0.99966309", "-0.00000644", "-0.00000672", "-0.00000260", "-0.00000184", "-0.00000479", "-0.00001099", "-0.00001347", "-0.00001280"], ["0.99898257", "0.99898369", "0.00000634", "0.00000730", "0.00000207", "0.00000360", "-0.00000002", "0.00000074", "0.00000350", "0.00000436"], ["-", "-", "0.00000324", "0.00000114", "0.00000174", "0.00000069", "-0.00001028", "-0.00001123", "-0.00001514", "-0.00001867"], ["1.00729492", "1.00730414", "0.00021279", "0.00043786", "0.00000024", "0.00003009", "0.00005593", "0.00011706", "0.00017152", "0.00022235"], ["1.00963793", "1.00965757", "0.00028601", "0.00062313", "-0.00000801", "0.00003538", "0.00007553", "0.00015793", "0.00026760", "0.00037069"], ["1.00040400", "1.00044298", "0.00029371", "0.00059574", "0.00000219", "0.00003805", "0.00007524", "0.00016661", "0.00024595", "0.00031366"], ["-", "-", "0.00079250", "0.00165672", "-0.00000558", "0.00010352", "0.00020671", "0.00044160", "0.00068507", "0.00090671"]] ("Test Data table")) -> ()
        }
        frame Enabled {
        }
      }
      n107 = call "SUB_Delay ms.vi"("delay(ms)"=u32 100 ("ms 타이머 값")) -> ()  [unwired: 3 in]
    }
    frame #5 {
      # "메인 루프"
      n108 = while {
        i -> [w249]
        stop <- w251 stop-if-true
        n109 = stacked-sequence {
          tunnel: w249 -> [_ w317 _ _ _ _ _ _ _ _ _ _]
          frame #0 {
            # "통신 연결 관리 - BLE"
            n110 = local read "Port close 1"() -> (w252:bool)
            n111 = local read "Port open 1"() -> (w253:bool)
            n112 = case shown="참" w253 {
              frame False {
              }
              frame True {
                # "통신 연결"
                n113 = stacked-sequence {
                  frame #0 {
                    # "초기화"
                    n114 = global write "Global 1.vi" "BLE Packet (buf)"(u8[] [] ("BLE Packet (buf)")) -> ()
                    n115 = global write "Global 1.vi" "BLE Packet (data)"(u8[][] [] ("BLE Packet (data)")) -> ()
                    n116 = global write "Global 1.vi" "BLE Packet"(FALSE ("BLE Packet")) -> ()
                    n117 = Tick Count (ms)() -> (millisecond timer value=w256:u32)
                    n118 = local write "ACT-Comm"(TRUE ("ACT-RS422")) -> ()
                    n119 = local write "Full ROM data"(FALSE ("Full ROM data")) -> ()
                    n120 = Initialize Array(T14 {"RxOK"=FALSE, "ROM Data"=[], "Index"=0} ("클러스터"), 32 ("차원 크기")) -> (w262:T10)
                    n121 = local write "Port open 1"(FALSE) -> ()
                    n122 = local write "Data trx(led)"(TRUE ("Rx")) -> ()
                    n123 = local write "Rx ROM-log"("" ("문자열-Rx ROM")) -> ()
                    n124 = local write "Timer-ble log"(w256) -> ()
                    n125 = local write "ROM Data"(w262) -> ()
                    n126 = local write "status string"("Communication connection attempt.." ("status string")) -> ()
                  }
                  frame #1 {
                    n127 = local read "Port-set 1"() -> (w267:refnum<visa-resource-name>)
                    n128 = call "_시리얼 포트-초기화.vi"("baud rate"=u32 115200, "시리얼 포트"=w267) -> ("정상"=w269:bool)  [unwired: 2 in, 1 out]
                    n129 = local write "Port-act 1"(w267) -> ()
                    n130 = case shown="거짓" w269 {
                      tunnel: w267 -> [_ w278]
                      frame False {
                        n131 = local write "Comm con status 1"(FALSE ("Connected")) -> ()
                        n132 = local write "Comm con 1"(FALSE ("보드 통신 연결 1")) -> ()
                        n133 = local write "Rx-mon"(TRUE ("수신 실패(T) 2")) -> ()
                        n134 = local write "RxD"("Can not find COM port" ("status string")) -> ()
                      }
                      frame True {
                        n135 = call "SUB-BLE SCAN.vi"("Port-set 1"=w278) -> ("Device Name"=→"Device Name":string, "Connection Status"=w274:T4, "Connected"=w277:bool)  [unwired: 2 in]
                        "Connection Status" <- w274
                        n136 = Not(x=w277) -> (.not. x?=w276:bool)
                        n137 = local write "Rx-mon"(w276) -> ()
                        n138 = case shown="거짓" w276 {
                          tunnel: w274 -> [_ w285]
                          frame True {
                            # "수신 데이터 에러 상태"
                            n139 = local read "Port-act 1"() -> (w282:refnum<visa-resource-name>)
                            n140 = VISA Close(VISA resource name=w282) -> ()  [unwired: 1 in, 1 out]
                            n141 = local write "Comm con status 1"(FALSE ("Connected")) -> ()
                            n142 = local write "*Board ID1"("None...." ("*Board ID")) -> ()
                            n143 = local write "Comm con 1"(FALSE ("보드 통신 연결 1")) -> ()
                            n144 = local write "Rx-mon"(TRUE ("수신 실패(T) 2")) -> ()
                          }
                          frame False {
                            w287 = T8 {"Left Wing-A, C1/C0"=0.0, "Left Wing-B, C2/C0"=0.0, "Left Wing-C, C3/C0"=0.0, "Right Wing-A, C4/C0"=0.0, "Right Wing-B, C5/C0"=0.0, "Right Wing-C, C6/C0"=0.0} ("CDC data")
                            w286 = T9 {"Gyroscope X"=0.0, "Gyroscope Y"=0.0, "Gyroscope Z"=0.0, "Accelerometer X"=0.0, "Accelerometer Y"=0.0, "Accelerometer Z"=0.0} ("IMU data")
                            # "수신 데이터 정상"
                            n145 = flat-sequence {
                              tunnel: w285 -> [w297]
                              tunnel: [w297] -> w284
                              tunnel: w284 -> [w298]
                              frame #0 {
                                n146 = Wait Until Next ms Multiple(millisecond multiple=u32 500 ("ms 타이머 값")) -> ()  [unwired: 1 out]
                              }
                              frame #1 {
                                # "데이터 전송\n- 핸들/0x01"
                                n147 = local read "Port-act 1"() -> (w302:refnum<visa-resource-name>)
                                n148 = String To Byte Array(string="\u0001" ("문자열")) -> (unsigned byte array=w300:u8[])
                                n149 = call-poly "ble_write_by_handle.vi"("Connection Status"=w298, "Handle"=u16 12, "data (uint8array)"=w300, "COM Bluegiga in"=w302) -> ()  [unwired: 6 in, 2 out]
                              }
                            }
                            n150 = local write "*Board ID1"("" ("*Board ID")) -> ()
                            n151 = local write "RxD"("Connection. OK....." ("status string")) -> ()
                            n152 = local write "Setting load(led)"(FALSE ("Power On Flag")) -> ()
                            n153 = local write "Comm con status 1"(TRUE ("Connected")) -> ()
                            n154 = local write "Comm err cnt 1"(0 ("통신에러카운트")) -> ()
                            n155 = local write "Clear graph 1"(TRUE ("그래프 지우기")) -> ()
                            n156 = local write "Clear graph 2"(TRUE ("그래프 지우기")) -> ()
                            n157 = local write "Comm con 1"(TRUE ("포트 연결")) -> ()
                            n158 = local write "CDC Offet"(w287) -> ()
                            n159 = local write "IMU data"(w286) -> ()
                            n160 = local write "IMU Offet"(w286) -> ()
                            n161 = local write "CDC data"(w287) -> ()
                          }
                        }
                      }
                    }
                  }
                  frame #2 {
                    n162 = local write "ACT-Comm"(FALSE ("ACT-RS422")) -> ()
                    n163 = local write "Data trx(led)"(FALSE ("Rx")) -> ()
                  }
                }
              }
            }
            n164 = case shown="참" w252 {
              frame False {
              }
              frame True {
                # "BLE 통신 종료"
                # "포트 닫기"
                n165 = local write "Port close 1"(FALSE ("포트닫기 1")) -> ()
                n166 = local write "Comm con status 1"(FALSE ("Connected")) -> ()
                n167 = local write "ACT-Comm"(FALSE ("ACT-RS422")) -> ()
                n168 = local write "status string"("Close communication port." ("status string")) -> ()
                n169 = local write "*Board ID1"("None...." ("*Board ID")) -> ()
                n170 = local write "Comm con 1"(FALSE ("보드 통신 연결 1")) -> ()
                n171 = local read "Port-act 1"() -> (w305:refnum<visa-resource-name>)
                n172 = local read "Connection Status"() -> (w310:T4)
                n173 = call "_시리얼_buf clear.vi"("시리얼 포트"=w305) -> ("에러 출력"=w308:errorcluster, "시리얼 포트 2"=w309:refnum<visa-resource-name>)  [unwired: 3 in]
                n174 = call "ble_disconnect_device.vi"("Connection Status"=w310, "error in (no error)"=w308, "COM Bluegiga in"=w309) -> ("error out"=w307:errorcluster, "COM Bluegiga out"=w306:refnum<visa-resource-name>)  [unwired: 7 in]
                n175 = VISA Close(VISA resource name=w306, error in (no error)=w307) -> ()  [unwired: 1 out]
              }
            }
          }
          frame #1 {
            # "BLE 수신 패킷 데이터 처리"
            n176 = local read "Comm con status 1"() -> (w318:bool)
            n177 = case shown="참" w318 {
              tunnel: w317 -> [_ w322]
              frame False {
              }
              frame True {
                w325 = 80 ("y")
                n178 = call "SUB-BLE Rx data Classify.vi"() -> ("data out"=w321:u8[], "Rx-set"=w319:bool, "Rx-mon"=w320:bool)  [unwired: 3 in]
                n179 = case shown="참" w320 {
                  tunnel: w321 -> [w329 w361]
                  tunnel: w319 -> [w328 _]
                  frame False {
                    # "초기 데이터"
                    n180 = local write "Rx-mon"(FALSE ("수신 실패(T) 1")) -> ()
                    n181 = case shown="참" w328 {
                      tunnel: w329 -> [_ w353]
                      frame False {
                      }
                      frame True {
                        # "데이터 입력 상태 체크"
                        n182 = call "SUB-BLE Rx data-ROM.vi"("data in"=w353) -> ("data Out"=w337:u8[], "Index"=w338:u8)  [unwired: 3 in]
                        n183 = local write "Rx-ROM"(TRUE ("Rx-ROM")) -> ()
                        n184 = property on="ROM Data" class="Arr (엄격한)"("Index Values"=u32[] [] ("인덱스 값")) -> ()  [unwired: 2 in, 2 out]
                        n185 = local read "ROM Data"() -> (w352:T10)
                        n186 = Bundle By Name(cluster=T14 {"RxOK"=FALSE, "ROM Data"=[], "Index"=0} ("클러스터"), "RxOK"=TRUE ("Packet Detect"), "ROM Data"=w337, "Index"=w338) -> (w350:T14)
                        n187 = Replace Array Subset(array=w352, new element=w350, index=w338) -> (w335:T10)
                        n188 = local read "Rx ROM-log"() -> (w346:string)
                        n189 = for {
                          tunnel: w335 -> [w355] mode=indexing
                          tunnel: [w354] -> w334 mode=indexing
                          n190 = Unbundle By Name(w355) -> ("RxOK"=w354:bool)
                        }
                        n191 = local write "ROM Data"(w335) -> ()
                        n192 = Format Into String(format string="%02d  " ("포맷 문자열"), w338) -> (resulting string=w340:string)  [unwired: 2 in, 1 out]
                        n193 = call <vilib>:"Space Constant.vi"() -> ("String"=w339:string)
                        n194 = Array To Spreadsheet String(delimiter (Tab)=w339, array=w337, 3:"%02X" ("포맷 문자열")) -> (spreadsheet string=w342:string)
                        n195 = Format Date/Time String(time format string (%c)="%H:%M:%S%3u>  " ("상태")) -> (date/time string=w344:string)  [unwired: 2 in]
                        n196 = Boolean Array To Number(Boolean array=w334) -> (number=w333:u32)
                        n197 = Concatenate Strings(w346, w340, w344, w342) -> (w345:string)
                        n198 = Equal?(x=w333, y=u32 4294967295) -> (x = y?=w332:bool)
                        n199 = local write "Full ROM data"(w332) -> ()
                        n200 = local write "Rx ROM-log"(w345) -> ()
                      }
                    }
                  }
                  frame True {
                    # "모니터링 데이터"
                    # "모니터링 데이터 수신 완료"
                    n201 = local write "Rx-mon"(TRUE ("Rx-mon")) -> ()
                    n202 = local write "Rx-ROM"(FALSE ("Rx-ROM")) -> ()
                    n203 = local read "ms timer"() -> (w370:u32)
                    n204 = Tick Count (ms)() -> (millisecond timer value=w369:u32)
                    n205 = call <vilib>:"Space Constant.vi"() -> ("String"=w364:string)
                    n206 = Subtract(x=w369, y=w370) -> (x-y=w367:u32)
                    n207 = Array To Spreadsheet String(delimiter (Tab)=w364, array=w361, 3:"%02X" ("포맷 문자열")) -> (spreadsheet string=w362:string)
                    n208 = local write "BLE Packet (mon)"(w361) -> ()
                    n209 = local write "ms timer"(w369) -> ()
                    n210 = local write "status string"("Receive a monitoring data..." ("status string")) -> ()
                    n211 = Format Into String(format string="[%d ms] " ("포맷 문자열"), w367) -> (resulting string=w366:string)  [unwired: 2 in, 1 out]
                    n212 = local read "ms timer 2"() -> (w358:u32)
                    n213 = Tick Count (ms)() -> (millisecond timer value=w357:u32)
                    n214 = Concatenate Strings(w366, w362) -> (w365:string)
                    n215 = Subtract(x=w357, y=w358) -> (x-y=w356:u32)
                    n216 = case shown="150.." w356 {
                      tunnel: w365 -> [_ w373]
                      frame 0, Default {
                      }
                      frame 150.. {
                        n217 = Tick Count (ms)() -> (millisecond timer value=w372:u32)
                        n218 = local write "RxD"(w373) -> ()
                        n219 = local write "ms timer 2"(w372) -> ()
                      }
                    }
                  }
                }
                n220 = Quotient & Remainder(x=w322, y=w325) -> (x-y*floor(x/y)=w323:i32)  [unwired: 1 out]
                n221 = Divide(x=w325, y=2) -> (x/y=w326:dbl)
                n222 = Greater?(x=w323, y=w326) -> (0:w324:bool)
                n223 = local write "ACT-Comm"(w324) -> ()
              }
            }
          }
          frame #2 {
            # "모니터링 데이터"
            n224 = local read "Rx-mon"() -> (w374:bool)
            n225 = case shown="참" w374 {
              frame False {
              }
              frame True {
                # "수신 데이터 처리"
                n226 = local read "ms timer 3"() -> (w379:u32)
                n227 = local read "Interval(ms)"() -> (w375:u16)
                n228 = Tick Count (ms)() -> (millisecond timer value=w378:u32)
                n229 = Subtract(x=w378, y=w379) -> (x-y=w376:u32)
                n230 = Greater Or Equal?(x=w376, y=w375) -> (x >= y?=w377:bool)
                n231 = case shown="참" w377 {
                  frame False {
                  }
                  frame True {
                    n232 = local read "BLE Packet (mon)"() -> (w384:u8[])
                    n233 = call "SUB-BLE Rx data-CDC IMU.vi"("data in"=w384) -> ("IMU data"=w381:T9, "CDC data"=w382:T8, "Bat"=w380:u16, "*Board ID"=w383:string)  [unwired: 4 in]
                    n234 = stacked-sequence {
                      seq-local: [w387 _ _ _ _ _] -> [_ _ w430 _ w461 _]
                      tunnel: w383 -> [w386 _ _ _ _ _]
                      tunnel: w382 -> [_ w401 _ _ _ _]
                      tunnel: w381 -> [_ _ _ w445 _ _]
                      tunnel: w380 -> [_ _ _ _ _ w483]
                      frame #0 {
                        # "SN"
                        n235 = Tick Count (ms)() -> (millisecond timer value=w385:u32)
                        n236 = local write "ms timer 3"(w385) -> ()
                        n237 = local write "*Board ID1"(w386) -> ()
                        n238 = local read "Graph timer 1"() -> (w388:u32)
                        n239 = Tick Count (ms)() -> (millisecond timer value=w389:u32)
                        n240 = flat-sequence {
                          tunnel: w389 -> [w394]
                          tunnel: w388 -> [w391]
                          tunnel: [w390] -> w387
                          frame #0 {
                            n241 = Subtract(x=w394, y=w391) -> (x-y=w392:u32)
                            n242 = local write "Graph timer 1"(w394) -> ()
                            n243 = Multiply(x=w392, y=0.001 ("dt")) -> (x*y=w390:dbl)
                          }
                        }
                      }
                      frame #1 {
                        # "CDC 데이터"
                        n244 = local read "CDC Offet"() -> (w416:T8)
                        n245 = Unbundle By Name(w401) -> ("Left Wing-A, C1/C0"=w400:dbl, "Left Wing-B, C2/C0"=w399:dbl, "Left Wing-C, C3/C0"=w398:dbl, "Right Wing-A, C4/C0"=w397:dbl, "Right Wing-B, C5/C0"=w396:dbl, "Right Wing-C, C6/C0"=w395:dbl)
                        n246 = Unbundle By Name(w416) -> ("Left Wing-A, C1/C0"=w415:dbl, "Left Wing-B, C2/C0"=w414:dbl, "Left Wing-C, C3/C0"=w413:dbl, "Right Wing-A, C4/C0"=w412:dbl, "Right Wing-B, C5/C0"=w411:dbl, "Right Wing-C, C6/C0"=w410:dbl)
                        n247 = Subtract(x=w400, y=w415) -> (x-y=w407:dbl)
                        n248 = Subtract(x=w399, y=w414) -> (x-y=w406:dbl)
                        n249 = Subtract(x=w398, y=w413) -> (x-y=w405:dbl)
                        n250 = Subtract(x=w397, y=w412) -> (x-y=w404:dbl)
                        n251 = Subtract(x=w396, y=w411) -> (x-y=w403:dbl)
                        n252 = Subtract(x=w395, y=w410) -> (x-y=w402:dbl)
                        n253 = local read "CDC data"() -> (w409:T8)
                        n254 = Bundle By Name(cluster=w409, "Left Wing-A, C1/C0"=w407, "Left Wing-B, C2/C0"=w406, "Left Wing-C, C3/C0"=w405, "Right Wing-A, C4/C0"=w404, "Right Wing-B, C5/C0"=w403, "Right Wing-C, C6/C0"=w402) -> (w408:T8)
                        n255 = local write "CDC data"(w408) -> ()
                      }
                      frame #2 {
                        # "* 그래프 출력"
                        n256 = local read "CDC data"() -> (w429:T8)
                        n257 = Unbundle By Name(w429) -> ("Left Wing-A, C1/C0"=w428:dbl, "Left Wing-B, C2/C0"=w421:dbl, "Left Wing-C, C3/C0"=w420:dbl, "Right Wing-A, C4/C0"=w419:dbl, "Right Wing-B, C5/C0"=w418:dbl, "Right Wing-C, C6/C0"=w417:dbl)
                        n258 = Build Array(w428) -> (w427:dbl[])
                        n259 = Get Date/Time In Seconds() -> (seconds since 1Jan1904=w433:timestamp)
                        n260 = Build Array(w421) -> (w426:dbl[])
                        n261 = Build Array(w420) -> (w425:dbl[])
                        n262 = Build Array(w418) -> (w423:dbl[])
                        n263 = Build Array(w419) -> (w424:dbl[])
                        n264 = Build Array(w417) -> (w422:dbl[])
                        n265 = Bundle By Name("t0"=w433, "Y"=w427, "dt"=w430) -> (w438:waveform(dbl))  [unwired: 1 in]
                        n266 = Bundle By Name("t0"=w433, "Y"=w426, "dt"=w430) -> (w437:waveform(dbl))  [unwired: 1 in]
                        n267 = Bundle By Name("t0"=w433, "Y"=w425, "dt"=w430) -> (w436:waveform(dbl))  [unwired: 1 in]
                        n268 = Bundle By Name("t0"=w433, "Y"=w424, "dt"=w430) -> (w434:waveform(dbl))  [unwired: 1 in]
                        n269 = Bundle By Name("t0"=w433, "Y"=w423, "dt"=w430) -> (w432:waveform(dbl))  [unwired: 1 in]
                        n270 = Bundle By Name("t0"=w433, "Y"=w422, "dt"=w430) -> (w431:waveform(dbl))  [unwired: 1 in]
                        n271 = Build Array(w438, w437, w436, w434, w432, w431) -> (→"CDC(PCAP02) Graph":waveform(dbl)[])
                      }
                      frame #3 {
                        # "IMU Data"
                        n272 = local read "IMU Offet"() -> (w460:T9)
                        n273 = Unbundle By Name(w445) -> ("Gyroscope X"=w444:dbl, "Gyroscope Y"=w443:dbl, "Gyroscope Z"=w442:dbl, "Accelerometer X"=w441:dbl, "Accelerometer Y"=w440:dbl, "Accelerometer Z"=w439:dbl)
                        n274 = Unbundle By Name(w460) -> ("Gyroscope X"=w457:dbl, "Gyroscope Y"=w456:dbl, "Gyroscope Z"=w455:dbl, "Accelerometer X"=w454:dbl, "Accelerometer Y"=w453:dbl, "Accelerometer Z"=w452:dbl)
                        n275 = Subtract(x=w444, y=w457) -> (x-y=w451:dbl)
                        n276 = Subtract(x=w443, y=w456) -> (x-y=w450:dbl)
                        n277 = Subtract(x=w442, y=w455) -> (x-y=w449:dbl)
                        n278 = Subtract(x=w441, y=w454) -> (x-y=w448:dbl)
                        n279 = Subtract(x=w440, y=w453) -> (x-y=w447:dbl)
                        n280 = Subtract(x=w439, y=w452) -> (x-y=w446:dbl)
                        n281 = local read "IMU data"() -> (w459:T9)
                        n282 = Bundle By Name(cluster=w459, "Gyroscope X"=w451, "Gyroscope Y"=w450, "Gyroscope Z"=w449, "Accelerometer X"=w448, "Accelerometer Y"=w447, "Accelerometer Z"=w446) -> (w458:T9)
                        n283 = local write "IMU data"(w458) -> ()
                      }
                      frame #4 {
                        # "* 그래프 출력"
                        n284 = local read "IMU data"() -> (w474:T9)
                        n285 = Unbundle By Name(w474) -> ("Gyroscope X"=w473:dbl, "Gyroscope Y"=w466:dbl, "Gyroscope Z"=w465:dbl, "Accelerometer X"=w464:dbl, "Accelerometer Y"=w463:dbl, "Accelerometer Z"=w462:dbl)
                        n286 = Build Array(w473) -> (w472:dbl[])
                        n287 = Get Date/Time In Seconds() -> (seconds since 1Jan1904=w477:timestamp)
                        n288 = Build Array(w466) -> (w471:dbl[])
                        n289 = Build Array(w465) -> (w470:dbl[])
                        n290 = Build Array(w463) -> (w468:dbl[])
                        n291 = Build Array(w464) -> (w469:dbl[])
                        n292 = Build Array(w462) -> (w467:dbl[])
                        n293 = Bundle By Name("t0"=w477, "Y"=w472, "dt"=w461) -> (w481:waveform(dbl))  [unwired: 1 in]
                        n294 = Bundle By Name("t0"=w477, "Y"=w471, "dt"=w461) -> (w480:waveform(dbl))  [unwired: 1 in]
                        n295 = Bundle By Name("t0"=w477, "Y"=w470, "dt"=w461) -> (w479:waveform(dbl))  [unwired: 1 in]
                        n296 = Bundle By Name("t0"=w477, "Y"=w469, "dt"=w461) -> (w478:waveform(dbl))  [unwired: 1 in]
                        n297 = Bundle By Name("t0"=w477, "Y"=w468, "dt"=w461) -> (w476:waveform(dbl))  [unwired: 1 in]
                        n298 = Bundle By Name("t0"=w477, "Y"=w467, "dt"=w461) -> (w475:waveform(dbl))  [unwired: 1 in]
                        n299 = Build Array(w481, w480, w479, w478, w476, w475) -> (→"IMU Graph":waveform(dbl)[])
                      }
                      frame #5 {
                        # "BAT raw data"
                        n300 = local write "Bat(raw)"(w483) -> ()
                      }
                    }
                  }
                }
              }
            }
          }
          frame #3 {
            # "Force Test"
            n301 = local read "Test Start"() -> (w484:bool)
            n302 = local read "Rx-mon"() -> (w485:bool)
            n303 = case shown="참" w485 {
              tunnel: w484 -> [_ w489]
              frame False {
                n304 = local write "FTS Testing"(FALSE ("FTS 시험 진행")) -> ()
                n305 = local write "FTS comm."(FALSE ("FTS 수신 정상")) -> ()
                n306 = local write "Test Start"(FALSE ("Test Start")) -> ()
              }
              frame True {
                n307 = case shown="참" w489 {
                  frame False {
                  }
                  frame True {
                    n308 = stacked-sequence {
                      frame #0 {
                        # "세로"
                        # "초기화"
                        n309 = Wait Until Next ms Multiple(millisecond multiple=u32 100 ("ms 배수")) -> ()  [unwired: 1 out]
                        n310 = for {
                          N: 9 -> [_]
                          tunnel: [w501] -> w493 mode=indexing
                          # "가로"
                          n311 = for {
                            N: 10 -> [_]
                            tunnel: ["-"] -> w501 mode=indexing
                          }
                        }
                        n312 = local write "Mark10 Gauge (lb)"(0.0 ("Mark10 Gauge")) -> ()
                        n313 = local write "FTS Testing"(TRUE ("FTS 시험 진행")) -> ()
                        n314 = local write "FTS comm."(FALSE ("FTS 수신 정상")) -> ()
                        n315 = local write "status string"("Force Test Mode..." ("status string")) -> ()
                        n316 = local write "FTS OP status"(T6 "시험 시작" ("FTS 동작시험 상태")) -> ()
                        n317 = Format Date/Time String(time format string (%c)="%Y/%m/%d %H:%M:%S> Force Test Start\n" ("상태")) -> (date/time string=w491:string)  [unwired: 2 in]
                        n318 = local write "Test Data table"(w493) -> ()
                        n319 = local write "Test Status"(w491) -> ()
                        n320 = local write "Load vs Ratio Graph"(cluster{dbl[], dbl[]}[] [] ("Load vs Ratio Graph")) -> ()
                      }
                      frame #1 {
                        n321 = local read "Port-FTS"() -> (w509:refnum<visa-resource-name>)
                        n322 = control-ref of="Test Status"() -> (w505:refnum<vi>)
                        n323 = call "_시리얼_Mark10-연결확인.vi"("시리얼 포트"=w509) -> ("수신 정상"=w508:bool, "VISA resource name out"=w507:refnum<visa-resource-name>)  [unwired: 3 in]
                        n324 = call "SUB-Status string update.vi"("텍스트 입력"="Check Serial port of Mark-10\n" ("Force Test Status"), "날짜추가"=TRUE, "reference"=w505) -> ()  [unwired: 2 in, 1 out]
                        n325 = case shown="거짓" w508 {
                          tunnel: w507 -> [_ _]
                          frame False {
                            # "통신 불량"
                            n326 = local write "FTS OP status"(T6 "시험 종료" ("FTS 동작시험 상태")) -> ()
                            n327 = One Button Dialog(message="Cannot find MARK10.\nCheck comm port." ("메시지")) -> ()  [unwired: 1 in, 1 out]
                          }
                          frame True {
                          }
                        }
                        n328 = local write "FTS comm."(w508) -> ()
                      }
                      frame #2 {
                        n329 = while {
                          stop <- w514 stop-if-true
                          # "시험 프로파일"
                          n330 = local read "FTS OP status"() -> (w515:T6)
                          n331 = local read "Test profile"() -> (w512:string[][])
                          n332 = Wait Until Next ms Multiple(millisecond multiple=u32 500 ("ms 배수")) -> ()  [unwired: 1 out]
                          n333 = case shown="\"시험 진행-압력시험\"" w515 {
                            tunnel: [w520 _ _ _ _ TRUE] -> w514
                            tunnel: w512 -> [_ _ _ w590 _ _]
                            frame "시험 시작" {
                              n334 = control-ref of="Test Status"() -> (w517:refnum<vi>)
                              n335 = local write "FTS OP status"(T6 "시험전 점검" ("FTS 동작시험 상태")) -> ()
                              n336 = call "SUB-Status string update.vi"("텍스트 입력"="Force Test Start!\n" ("Force Test Status"), "날짜추가"=TRUE, "reference"=w517) -> ()  [unwired: 2 in, 1 out]
                              n337 = local read "stop"() -> (w520:bool)
                            }
                            frame "시험전 점검" {
                              n338 = local read "Port-FTS"() -> (w522:refnum<visa-resource-name>)
                              n339 = call "_시리얼_Mark10-데이터 수신 (게이지).vi"("시리얼 포트"=w522) -> ("데이터(lb)"=w521:dbl, "수신 정상"=w523:bool)  [unwired: 2 in, 1 out]
                              n340 = local write "Mark10 Gauge (lb)"(w521) -> ()
                              n341 = local write "FTS comm."(w523) -> ()
                              n342 = local write "FTS OP status"(T6 "시험 진행-CDC 옵셋" ("FTS 동작시험 상태")) -> ()
                            }
                            frame "시험 진행-CDC 옵셋" {
                              n343 = stacked-sequence {
                                frame #0 {
                                n344 = control-ref of="Test Status"() -> (w526:refnum<vi>)
                                n345 = call "SUB-Status string update.vi"("텍스트 입력"="Offset data set... start" ("Force Test Status"), "날짜추가"=TRUE, "reference"=w526) -> ()  [unwired: 2 in, 1 out]
                                }
                                frame #1 {
                                n346 = Wait Until Next ms Multiple(millisecond multiple=u32 500 ("ms 배수")) -> ()  [unwired: 1 out]
                                }
                                frame #2 {
                                n347 = for {
                                N: 50 -> [_]
                                tunnel: [w551] -> w542 mode=indexing
                                tunnel: [w550] -> w541 mode=indexing
                                tunnel: [w549] -> w540 mode=indexing
                                tunnel: [w548] -> w539 mode=indexing
                                tunnel: [w547] -> w538 mode=indexing
                                tunnel: [w546] -> w537 mode=indexing
                                n348 = local read "CDC Offet"() -> (w544:T8)
                                n349 = local read "Test Status"() -> (w556:string)
                                n350 = call "SUB-BLE Rx Wait.vi"("Timeout(ms)"=u16 200) -> ("RxReady"=w552:bool)  [unwired: 4 in]
                                n351 = case shown="참" w552 {
                                tunnel: [w558 w559] -> w545
                                tunnel: w544 -> [w558 _]
                                frame False {
                                }
                                frame True {
                                n352 = call "SUB-BLE Rx data Classify.vi"() -> ("data out"=w560:u8[])  [unwired: 3 in, 2 out]
                                n353 = call "SUB-BLE Rx data-CDC IMU.vi"("data in"=w560) -> ("CDC data"=w559:T8)  [unwired: 4 in, 3 out]
                                }
                                }
                                n354 = Concatenate Strings(w556, ".") -> (w557:string)
                                n355 = local write "Test Status"(w557) -> ()
                                n356 = Unbundle By Name(w545) -> ("Left Wing-A, C1/C0"=w551:dbl, "Left Wing-B, C2/C0"=w550:dbl, "Left Wing-C, C3/C0"=w549:dbl, "Right Wing-A, C4/C0"=w548:dbl, "Right Wing-B, C5/C0"=w547:dbl, "Right Wing-C, C6/C0"=w546:dbl)
                                n357 = Wait Until Next ms Multiple(millisecond multiple=u32 20 ("ms 배수")) -> ()  [unwired: 1 out]
                                }
                                n358 = call-poly <vilib>:"Mean.vi"("X"=w542) -> ("mean"=w534:dbl)  [unwired: 1 out]
                                n359 = call-poly <vilib>:"Mean.vi"("X"=w541) -> ("mean"=w533:dbl)  [unwired: 1 out]
                                n360 = call-poly <vilib>:"Mean.vi"("X"=w540) -> ("mean"=w532:dbl)  [unwired: 1 out]
                                n361 = call-poly <vilib>:"Mean.vi"("X"=w539) -> ("mean"=w531:dbl)  [unwired: 1 out]
                                n362 = call-poly <vilib>:"Mean.vi"("X"=w538) -> ("mean"=w530:dbl)  [unwired: 1 out]
                                n363 = call-poly <vilib>:"Mean.vi"("X"=w537) -> ("mean"=w529:dbl)  [unwired: 1 out]
                                n364 = Bundle By Name(cluster=T8 {"Left Wing-A, C1/C0"=0.0, "Left Wing-B, C2/C0"=0.0, "Left Wing-C, C3/C0"=0.0, "Right Wing-A, C4/C0"=0.0, "Right Wing-B, C5/C0"=0.0, "Right Wing-C, C6/C0"=0.0} ("CDC data"), "Left Wing-A, C1/C0"=w534, "Left Wing-B, C2/C0"=w533, "Left Wing-C, C3/C0"=w532, "Right Wing-A, C4/C0"=w531, "Right Wing-B, C5/C0"=w530, "Right Wing-C, C6/C0"=w529) -> (w535:T8)
                                n365 = local write "CDC Offet"(w535) -> ()
                                }
                                frame #3 {
                                n366 = local read "Test Status"() -> (w562:string)
                                n367 = Concatenate Strings(w562, "\n") -> (w563:string)
                                n368 = local write "Test Status"(w563) -> ()
                                }
                                frame #4 {
                                w565 = "-"
                                w573 = i16 8 ("정밀도(6)")
                                n369 = local read "CDC Offet"() -> (w586:T8)
                                n370 = control-ref of="Test Status"() -> (w588:refnum<vi>)
                                n371 = Unbundle By Name(w586) -> ("Left Wing-A, C1/C0"=w585:dbl, "Left Wing-B, C2/C0"=w584:dbl, "Left Wing-C, C3/C0"=w583:dbl, "Right Wing-A, C4/C0"=w579:dbl, "Right Wing-B, C5/C0"=w578:dbl, "Right Wing-C, C6/C0"=w577:dbl)
                                n372 = local write "FTS OP status"(T6 "시험 진행-압력시험" ("FTS 동작시험 상태")) -> ()
                                n373 = call "SUB-Status string update.vi"("텍스트 입력"="Offset data set... done\n" ("Force Test Status"), "날짜추가"=TRUE, "reference"=w588) -> ()  [unwired: 2 in, 1 out]
                                n374 = local read "Mark10 Gauge (lb)"() -> (w567:dbl)
                                n375 = Number To Fractional String(number=w567, precision (6)=i16 2 ("정밀도(6)")) -> (F-format string=w564:string)  [unwired: 2 in]
                                n376 = Number To Fractional String(number=w585, precision (6)=w573) -> (F-format string=w582:string)  [unwired: 2 in]
                                n377 = Number To Fractional String(number=w584, precision (6)=w573) -> (F-format string=w581:string)  [unwired: 2 in]
                                n378 = Number To Fractional String(number=w583, precision (6)=w573) -> (F-format string=w580:string)  [unwired: 2 in]
                                n379 = Number To Fractional String(number=w579, precision (6)=w573) -> (F-format string=w576:string)  [unwired: 2 in]
                                n380 = Number To Fractional String(number=w578, precision (6)=w573) -> (F-format string=w575:string)  [unwired: 2 in]
                                n381 = Number To Fractional String(number=w577, precision (6)=w573) -> (F-format string=w574:string)  [unwired: 2 in]
                                n382 = local read "Test Data table"() -> (w570:string[][])
                                n383 = Build Array(w564, w582, w581, w580, w565, w576, w575, w574, w565) -> (w572:string[])
                                n384 = Replace Array Subset(array=w570, new element=w572, index (col)=0 ("비활성화된 인덱스 (열)")) -> (w571:string[][])  [unwired: 1 in]
                                n385 = local write "Test Data table"(w571) -> ()
                                }
                              }
                            }
                            frame "시험 진행-압력시험" {
                              n386 = stacked-sequence {
                                tunnel: w590 -> [_ w594 _ _]
                                frame #0 {
                                n387 = control-ref of="Test Status"() -> (w592:refnum<vi>)
                                n388 = call "SUB-Status string update.vi"("텍스트 입력"="Start Force test by Profile" ("Force Test Status"), "날짜추가"=TRUE, "reference"=w592) -> ()  [unwired: 2 in, 1 out]
                                }
                                frame #1 {
                                n389 = for {
                                tunnel: w594 -> [w596] mode=indexing
                                i -> [w597]
                                stop <- w595 continue-if-true
                                n390 = stacked-sequence {
                                tunnel: w597 -> [w601 _ _ w626 _ w723 w738]
                                tunnel: w596 -> [w600 w613 w617 _ _ _ _]
                                tunnel: [_ w608 _ _ _ _ _] -> w595
                                frame #0 {
                                # "진행 상태 문자열"
                                n391 = Index Array(array=w600, index=0 ("인덱스")) -> (element=w598:string)
                                n392 = Increment(x=w601) -> (x+1=w602:i32)
                                n393 = control-ref of="Test Status"() -> (w605:refnum<vi>)
                                n394 = Format Into String(format string="Force Testing-Profile(%d)...%s" ("Force Test Status"), w602, w598) -> (resulting string=w604:string)  [unwired: 2 in, 1 out]
                                n395 = call "SUB-Status string update.vi"("텍스트 입력"=w604, "날짜추가"=TRUE, "reference"=w605) -> ()  [unwired: 2 in, 1 out]
                                }
                                frame #1 {
                                # "압력 인가"
                                n396 = Index Array(array=w613, index=1 ("인덱스")) -> (element=w611:string)
                                n397 = local read "Port-FTS"() -> (w614:refnum<visa-resource-name>)
                                n398 = Fract/Exp String To Number(string=w611) -> (number=w610:dbl)  [unwired: 3 in, 1 out]
                                n399 = call "_시리얼_Mark10-제어 (압력설정).vi"("FTS 제어 상태"=T16 "압력제어 시작", "압력 설정(lb)"=w610, "시리얼 포트"=w614) -> ("게이지 압력(lb)"=w607:dbl, "통신 정상"=w608:bool)  [unwired: 1 out]
                                n400 = local write "Mark10 Gauge (lb)"(w607) -> ()
                                n401 = local write "FTS comm."(w608) -> ()
                                }
                                frame #2 {
                                # "대기 시간."
                                n402 = Tick Count (ms)() -> (millisecond timer value=w616:u32)
                                n403 = Index Array(array=w617, index=2 ("인덱스")) -> (element=w618:string)
                                n404 = Fract/Exp String To Number(string=w618) -> (number=w615:dbl)  [unwired: 3 in, 1 out]
                                n405 = while {
                                tunnel: w616 -> [w624]
                                tunnel: w615 -> [w622]
                                stop <- w621 stop-if-true
                                n406 = Tick Count (ms)() -> (millisecond timer value=w625:u32)
                                n407 = Subtract(x=w625, y=w624) -> (x-y=w623:u32)
                                n408 = Greater Or Equal?(x=w623, y=w622) -> (x >= y?=w621:bool)
                                n409 = Wait Until Next ms Multiple(millisecond multiple=u32 20 ("ms 배수")) -> ()  [unwired: 1 out]
                                }
                                }
                                frame #3 {
                                n410 = case shown="2" w626 {
                                frame 0, Default {
                                }
                                frame 2 {
                                n411 = stacked-sequence {
                                frame #0 {
                                # "Offset"
                                n412 = for {
                                N: 50 -> [_]
                                tunnel: [w649] -> w640 mode=indexing
                                tunnel: [w648] -> w639 mode=indexing
                                tunnel: [w647] -> w638 mode=indexing
                                tunnel: [w646] -> w637 mode=indexing
                                tunnel: [w645] -> w636 mode=indexing
                                tunnel: [w644] -> w635 mode=indexing
                                n413 = local read "CDC Offet"() -> (w642:T8)
                                n414 = call "SUB-BLE Rx Wait.vi"("Timeout(ms)"=u16 200) -> ("RxReady"=w650:bool)  [unwired: 4 in]
                                n415 = case shown="참" w650 {
                                tunnel: [w653 w654] -> w643
                                tunnel: w642 -> [w653 _]
                                frame False {
                                }
                                frame True {
                                n416 = call "SUB-BLE Rx data Classify.vi"() -> ("data out"=w655:u8[])  [unwired: 3 in, 2 out]
                                n417 = call "SUB-BLE Rx data-CDC IMU.vi"("data in"=w655) -> ("CDC data"=w654:T8)  [unwired: 4 in, 3 out]
                                }
                                }
                                n418 = Unbundle By Name(w643) -> ("Left Wing-A, C1/C0"=w649:dbl, "Left Wing-B, C2/C0"=w648:dbl, "Left Wing-C, C3/C0"=w647:dbl, "Right Wing-A, C4/C0"=w646:dbl, "Right Wing-B, C5/C0"=w645:dbl, "Right Wing-C, C6/C0"=w644:dbl)
                                n419 = Wait Until Next ms Multiple(millisecond multiple=u32 20 ("ms 배수")) -> ()  [unwired: 1 out]
                                }
                                n420 = call-poly <vilib>:"Mean.vi"("X"=w640) -> ("mean"=w632:dbl)  [unwired: 1 out]
                                n421 = call-poly <vilib>:"Mean.vi"("X"=w639) -> ("mean"=w631:dbl)  [unwired: 1 out]
                                n422 = call-poly <vilib>:"Mean.vi"("X"=w638) -> ("mean"=w630:dbl)  [unwired: 1 out]
                                n423 = call-poly <vilib>:"Mean.vi"("X"=w637) -> ("mean"=w629:dbl)  [unwired: 1 out]
                                n424 = call-poly <vilib>:"Mean.vi"("X"=w636) -> ("mean"=w628:dbl)  [unwired: 1 out]
                                n425 = call-poly <vilib>:"Mean.vi"("X"=w635) -> ("mean"=w627:dbl)  [unwired: 1 out]
                                n426 = Bundle By Name(cluster=T8 {"Left Wing-A, C1/C0"=0.0, "Left Wing-B, C2/C0"=0.0, "Left Wing-C, C3/C0"=0.0, "Right Wing-A, C4/C0"=0.0, "Right Wing-B, C5/C0"=0.0, "Right Wing-C, C6/C0"=0.0} ("CDC data"), "Left Wing-A, C1/C0"=w632, "Left Wing-B, C2/C0"=w631, "Left Wing-C, C3/C0"=w630, "Right Wing-A, C4/C0"=w629, "Right Wing-B, C5/C0"=w628, "Right Wing-C, C6/C0"=w627) -> (w633:T8)
                                n427 = local write "CDC Offet"(w633) -> ()
                                }
                                frame #1 {
                                w657 = "-"
                                w664 = i16 8 ("정밀도(6)")
                                n428 = local read "CDC Offet"() -> (w677:T8)
                                n429 = Unbundle By Name(w677) -> ("Left Wing-A, C1/C0"=w676:dbl, "Left Wing-B, C2/C0"=w675:dbl, "Left Wing-C, C3/C0"=w674:dbl, "Right Wing-A, C4/C0"=w670:dbl, "Right Wing-B, C5/C0"=w669:dbl, "Right Wing-C, C6/C0"=w668:dbl)
                                n430 = local read "Mark10 Gauge (lb)"() -> (w659:dbl)
                                n431 = local read "Test Data table"() -> (w661:string[][])
                                n432 = Number To Fractional String(number=w659, precision (6)=i16 2 ("정밀도(6)")) -> (F-format string=w656:string)  [unwired: 2 in]
                                n433 = Number To Fractional String(number=w676, precision (6)=w664) -> (F-format string=w673:string)  [unwired: 2 in]
                                n434 = Number To Fractional String(number=w675, precision (6)=w664) -> (F-format string=w672:string)  [unwired: 2 in]
                                n435 = Number To Fractional String(number=w674, precision (6)=w664) -> (F-format string=w671:string)  [unwired: 2 in]
                                n436 = Number To Fractional String(number=w670, precision (6)=w664) -> (F-format string=w667:string)  [unwired: 2 in]
                                n437 = Number To Fractional String(number=w669, precision (6)=w664) -> (F-format string=w666:string)  [unwired: 2 in]
                                n438 = Number To Fractional String(number=w668, precision (6)=w664) -> (F-format string=w665:string)  [unwired: 2 in]
                                n439 = Build Array(w656, w673, w672, w671, w657, w667, w666, w665, w657) -> (w663:string[])
                                n440 = Replace Array Subset(array=w661, new element=w663, index (col)=1 ("비활성화된 인덱스 (열)")) -> (w662:string[][])  [unwired: 1 in]
                                n441 = local write "Test Data table"(w662) -> ()
                                }
                                }
                                }
                                }
                                }
                                frame #4 {
                                # "CDC 데이터 수집"
                                n442 = for {
                                N: 10 -> [_]
                                tunnel: [w700] -> w691 mode=indexing
                                tunnel: [w699] -> w690 mode=indexing
                                tunnel: [w698] -> w689 mode=indexing
                                tunnel: [w697] -> w688 mode=indexing
                                tunnel: [w696] -> w687 mode=indexing
                                tunnel: [w695] -> w686 mode=indexing
                                n443 = local read "CDC data"() -> (w693:T8)
                                n444 = call "SUB-BLE Rx Wait.vi"("Timeout(ms)"=u16 200) -> ("RxReady"=w701:bool)  [unwired: 4 in]
                                n445 = case shown="참" w701 {
                                tunnel: [w704 w705] -> w694
                                tunnel: w693 -> [w704 _]
                                frame False {
                                }
                                frame True {
                                n446 = call "SUB-BLE Rx data Classify.vi"() -> ("data out"=w706:u8[])  [unwired: 3 in, 2 out]
                                n447 = call "SUB-BLE Rx data-CDC IMU.vi"("data in"=w706) -> ("CDC data"=w705:T8)  [unwired: 4 in, 3 out]
                                }
                                }
                                n448 = Unbundle By Name(w694) -> ("Left Wing-A, C1/C0"=w700:dbl, "Left Wing-B, C2/C0"=w699:dbl, "Left Wing-C, C3/C0"=w698:dbl, "Right Wing-A, C4/C0"=w697:dbl, "Right Wing-B, C5/C0"=w696:dbl, "Right Wing-C, C6/C0"=w695:dbl)
                                n449 = Wait Until Next ms Multiple(millisecond multiple=u32 20 ("ms 배수")) -> ()  [unwired: 1 out]
                                }
                                n450 = call-poly <vilib>:"Mean.vi"("X"=w691) -> ("mean"=w683:dbl)  [unwired: 1 out]
                                n451 = call-poly <vilib>:"Mean.vi"("X"=w690) -> ("mean"=w682:dbl)  [unwired: 1 out]
                                n452 = call-poly <vilib>:"Mean.vi"("X"=w689) -> ("mean"=w681:dbl)  [unwired: 1 out]
                                n453 = call-poly <vilib>:"Mean.vi"("X"=w688) -> ("mean"=w680:dbl)  [unwired: 1 out]
                                n454 = call-poly <vilib>:"Mean.vi"("X"=w687) -> ("mean"=w679:dbl)  [unwired: 1 out]
                                n455 = call-poly <vilib>:"Mean.vi"("X"=w686) -> ("mean"=w678:dbl)  [unwired: 1 out]
                                n456 = Bundle By Name(cluster=T8 {"Left Wing-A, C1/C0"=0.0, "Left Wing-B, C2/C0"=0.0, "Left Wing-C, C3/C0"=0.0, "Right Wing-A, C4/C0"=0.0, "Right Wing-B, C5/C0"=0.0, "Right Wing-C, C6/C0"=0.0} ("CDC data"), "Left Wing-A, C1/C0"=w683, "Left Wing-B, C2/C0"=w682, "Left Wing-C, C3/C0"=w681, "Right Wing-A, C4/C0"=w680, "Right Wing-B, C5/C0"=w679, "Right Wing-C, C6/C0"=w678) -> (w684:T8)
                                n457 = local write "CDC data"(w684) -> ()
                                }
                                frame #5 {
                                w719 = i16 8 ("정밀도(6)")
                                n458 = local read "CDC data"() -> (w733:T8)
                                n459 = Unbundle By Name(w733) -> ("Left Wing-A, C1/C0"=w714:dbl, "Left Wing-B, C2/C0"=w715:dbl, "Left Wing-C, C3/C0"=w716:dbl, "Right Wing-A, C4/C0"=w712:dbl, "Right Wing-B, C5/C0"=w711:dbl, "Right Wing-C, C6/C0"=w710:dbl)
                                n460 = local read "Mark10 Gauge (lb)"() -> (w709:dbl)
                                n461 = Compound Arithmetic op=ADD(w716, w715, w714) -> (w717:dbl)
                                n462 = Compound Arithmetic op=ADD(w712, w711, w710) -> (w713:dbl)
                                n463 = Number To Fractional String(number=w714, precision (6)=w719) -> (F-format string=w732:string)  [unwired: 2 in]
                                n464 = Number To Fractional String(number=w715, precision (6)=w719) -> (F-format string=w731:string)  [unwired: 2 in]
                                n465 = Number To Fractional String(number=w709, precision (6)=i16 2 ("정밀도(6)")) -> (F-format string=w707:string)  [unwired: 2 in]
                                n466 = Number To Fractional String(number=w716, precision (6)=w719) -> (F-format string=w730:string)  [unwired: 2 in]
                                n467 = Number To Fractional String(number=w717, precision (6)=w719) -> (F-format string=w720:string)  [unwired: 2 in]
                                n468 = Number To Fractional String(number=w712, precision (6)=w719) -> (F-format string=w729:string)  [unwired: 2 in]
                                n469 = Number To Fractional String(number=w711, precision (6)=w719) -> (F-format string=w728:string)  [unwired: 2 in]
                                n470 = Number To Fractional String(number=w710, precision (6)=w719) -> (F-format string=w727:string)  [unwired: 2 in]
                                n471 = Number To Fractional String(number=w713, precision (6)=w719) -> (F-format string=w718:string)  [unwired: 2 in]
                                n472 = local read "Test Data table"() -> (w724:string[][])
                                n473 = Build Array(w707, w732, w731, w730, w720, w729, w728, w727, w718) -> (w726:string[])
                                n474 = Add(x=2, y=w723) -> (x+y=w721:i32)
                                n475 = Replace Array Subset(array=w724, new element=w726, index (col)=w721) -> (w725:string[][])  [unwired: 1 in]
                                n476 = local write "Test Data table"(w725) -> ()
                                }
                                frame #6 {
                                # "로드 그래프"
                                n477 = local read "Test Data table"() -> (w745:string[][])
                                n478 = Subtract(x=w738, y=1 ("비활성화된 인덱스 (열)")) -> (x-y=w737:i32)
                                n479 = In Range and Coerce(upper limit=9 ("비활성화된 인덱스 (열)"), x=w737, lower limit=1 ("비활성화된 인덱스 (열)")) -> (coerced(x)=w735:i32)  [unwired: 1 out]
                                n480 = Array Subset(array=w745, index (col)=4 ("비활성화된 인덱스 (열)"), length (col)=w735) -> (w740:string[][])  [unwired: 2 in]
                                n481 = Fract/Exp String To Number(string=w740) -> (number=w744:dbl[][])  [unwired: 3 in, 1 out]
                                n482 = for {
                                N: 8 -> [_]
                                tunnel: [w753] -> w743 mode=indexing
                                tunnel: w744 -> [w752]
                                i -> [w750]
                                # "Y"
                                # "X"
                                n483 = Add(x=1, y=w750) -> (x+y=w748:i32)
                                n484 = Index Array(array=w752, index (row)=0 ("비활성화된 인덱스 (열)")) -> (element=w747:dbl[])  [unwired: 1 in]
                                n485 = Index Array(array=w752, index (row)=w748) -> (element=w746:dbl[])  [unwired: 1 in]
                                n486 = Bundle(w747, w746) -> (w753:cluster{dbl[], dbl[]})  [unwired: 1 in]
                                }
                                "Load vs Ratio Graph" <- w743
                                }
                                }
                                }
                                }
                                frame #2 {
                                n487 = local read "Port-FTS"() -> (w756:refnum<visa-resource-name>)
                                n488 = call "_시리얼_Mark10-제어 (압력설정).vi"("FTS 제어 상태"=T16 "헤더 상단 이동", "시리얼 포트"=w756) -> ("게이지 압력(lb)"=w754:dbl, "통신 정상"=w757:bool)  [unwired: 1 in, 1 out]
                                n489 = local write "Mark10 Gauge (lb)"(w754) -> ()
                                n490 = local write "FTS comm."(w757) -> ()
                                }
                                frame #3 {
                                n491 = control-ref of="Test Status"() -> (w759:refnum<vi>)
                                n492 = local write "FTS OP status"(T6 "시험 후 점검" ("FTS 동작시험 상태")) -> ()
                                n493 = call "SUB-Status string update.vi"("텍스트 입력"="Done Force test by Profile\n" ("Force Test Status"), "날짜추가"=TRUE, "reference"=w759) -> ()  [unwired: 2 in, 1 out]
                                }
                              }
                            }
                            frame "시험 후 점검" {
                              # "시험 종료 & \n측정 데이터 저장"
                              n494 = stacked-sequence {
                                seq-local: [_ w778 _ _ _] -> [_ _ _ _ w832]
                                seq-local: [_ _ w791 _ _] -> [_ _ _ _ w825]
                                seq-local: [_ _ _ w820 _] -> [_ _ _ _ w824]
                                seq-local: [_ _ _ w819 _] -> [_ _ _ _ w823]
                                seq-local: [w766 _ _ _ _] -> [_ w777 _ _ _]
                                frame #0 {
                                w774 = T24 1 items=["사용자 홈"=0, "사용자 데스크탑"=1, "사용자 문서"=2, "사용자 어플리케이션 데이터"=3, "사용자 환경"=4, "사용자 임시"=5, "퍼블릭 문서"=6, "퍼블릭 어플리케이션 데이터"=7, "퍼블릭 환경"=8, "퍼블릭 캐시"=13, "시스템 코어 라이브러리"=9, "시스템 설치된 라이브러리"=10, "어플리케이션 파일"=11, "부팅 볼륨 루트"=12] ("system directory type")
                                n495 = call <vilib>:"Get System Directory.vi"("system directory type"=w774) -> ("system directory"=w773:path)  [unwired: 10 in]
                                n496 = Path To String(path=w773) -> (string=w772:string)
                                n497 = Concatenate Strings(w772, "\\GEN4-GUI Test data" ("상태")) -> (w766:string)
                                n498 = String To Path(string=w766) -> (path=w770:path)
                                n499 = call <vilib>:"Check if File or Folder Exists.vi"("path"=w770) -> ("error out"=w767:errorcluster, "file or folder exists?"=w769:bool, "dup path"=w768:path)  [unwired: 8 in]
                                n500 = case shown="거짓" w769 {
                                tunnel: w768 -> [w776 _]
                                tunnel: w767 -> [w775 _]
                                frame False {
                                n501 = Create Folder(path (use dialog)=w776, error in=w775) -> ()  [unwired: 1 in, 3 out]
                                }
                                frame True {
                                }
                                }
                                }
                                frame #1 {
                                # "파일 저장 경로"
                                n502 = local read "Test name"() -> (w783:string)
                                n503 = Format Date/Time String(time format string (%c)="%Y%m%d %H%M%S" ("상태")) -> (date/time string=w782:string)  [unwired: 2 in]
                                n504 = Format Into String(format string="\\\\GEN4 Force Test-%s (%s).xlsx" ("상태"), w782, w783) -> (resulting string=w779:string)  [unwired: 2 in, 1 out]
                                n505 = Concatenate Strings(w777, w779) -> (w784:string)
                                n506 = String To Path(string=w784) -> (path=w778:path)
                                }
                                frame #2 {
                                # "remove sum data"
                                # "Fitting"
                                # "Y:인가압력"
                                n507 = local read "Test Data table"() -> (w806:string[][])
                                n508 = Fract/Exp String To Number(string=w806) -> (number=w800:dbl[][])  [unwired: 3 in, 1 out]
                                n509 = Delete From Array(array=w800, length=1 ("길이"), index (row)=4 ("인덱스 (행)")) -> (array with subset deleted=w795:dbl[][])  [unwired: 1 in, 1 out]
                                n510 = Delete From Array(array=w795, length=1 ("길이"), index (row)=7 ("인덱스 (행)")) -> (array with subset deleted=w790:dbl[][])  [unwired: 1 in, 1 out]
                                n511 = Array Subset(array=w790, index (col)=4 ("인덱스")) -> (w805:dbl[][])  [unwired: 3 in]
                                n512 = Array Subset(array=w790, index (row)=1 ("인덱스 (행)"), length (row)=6 ("인덱스 (행)")) -> (w787:dbl[][])  [unwired: 2 in]
                                n513 = Index Array(array=w805, index (row)=0 ("비활성화된 인덱스 (열)")) -> (element=w802:dbl[])  [unwired: 1 in]
                                n514 = Array Subset(array=w805, index (row)=1 ("인덱스")) -> (w803:dbl[][])  [unwired: 3 in]
                                n515 = Index Array(array=w787, index (col)=1 ("인덱스 (행)")) -> (element=w785:dbl[])  [unwired: 1 in]
                                n516 = for {
                                N: 6 -> [_]
                                tunnel: w803 -> [w818]
                                tunnel: w802 -> [w816]
                                tunnel: [w812] -> w794 mode=indexing
                                tunnel: w785 -> [_] mode=indexing
                                i -> [w813]
                                # "Offset"
                                # "X:CDC data"
                                n517 = Index Array(array=w818, index (row)=w813) -> (element=w811:dbl[])  [unwired: 1 in]
                                n518 = Add(x=w811, y=ext 0.0 ("polynomial order")) -> (x+y=w810:ext[])
                                n519 = Divide(x=w816, y=ext 3.0 ("polynomial order")) -> (x/y=w814:ext[])
                                n520 = call <vilib>:"General Polynomial Fit.vi"("Y"=w814, "polynomial order"=3, "X"=w810) -> ("Polynomial Coefficients"=w812:dbl[])  [unwired: 9 in, 3 out]
                                }
                                n521 = Number To Fractional String(number=w794, precision (6)=i16 15 ("정밀도(6)")) -> (F-format string=w792:string[][])  [unwired: 2 in]
                                n522 = Transpose 2D Array(2D array=w792) -> (transposed array=w791:string[][])
                                }
                                frame #3 {
                                # "column header"
                                # "row header"
                                # "Fotting Table - header"
                                n523 = call "SUB-module-여러줄 문자열을 배열로 변환.vi"("문자열"=" Coefficient X^0\nCoefficient X^1\nCoefficient X^2\nCoefficient X^3") -> ("배열"=w820:string[])
                                n524 = call "SUB-module-여러줄 문자열을 배열로 변환.vi"("문자열"="Left Wing-A\nLeft Wing-B\nLeft Wing-C\nRight Wing-A\nRight Wing-B\nRight Wing-C") -> ("배열"=w819:string[])
                                }
                                frame #4 {
                                w829 = 36 items=["xlRangeAutoFormat3DEffects1"=13, "xlRangeAutoFormat3DEffects2"=14, "xlRangeAutoFormatAccounting1"=4, "xlRangeAutoFormatAccounting2"=5, "xlRangeAutoFormatAccounting3"=6, "xlRangeAutoFormatAccounting4"=17, "xlRangeAutoFormatClassic1"=1, "xlRangeAutoFormatClassic2"=2, "xlRangeAutoFormatClassic3"=3, "xlRangeAutoFormatColor1"=7, "xlRangeAutoFormatColor2"=8, "xlRangeAutoFormatColor3"=9, "xlRangeAutoFormatList1"=10, "xlRangeAutoFormatList2"=11, "xlRangeAutoFormatList3"=12, "xlRangeAutoFormatLocalFormat1"=15, "xlRangeAutoFormatLocalFormat2"=16, "xlRangeAutoFormatLocalFormat3"=19, "xlRangeAutoFormatLocalFormat4"=20, "xlRangeAutoFormatReport1"=21, "xlRangeAutoFormatReport2"=22, "xlRangeAutoFormatReport3"=23, "xlRangeAutoFormatReport4"=24, "xlRangeAutoFormatReport5"=25, "xlRangeAutoFormatReport6"=26, "xlRangeAutoFormatReport7"=27, "xlRangeAutoFormatReport8"=28, "xlRangeAutoFormatReport9"=29, "xlRangeAutoFormatReport10"=30, "xlRangeAutoFormatClassicPivotTable"=31, "xlRangeAutoFormatTable1"=32, "xlRangeAutoFormatTable2"=33, "xlRangeAutoFormatTable3"=34, "xlRangeAutoFormatTable4"=35, "xlRangeAutoFormatTable5"=36, "xlRangeAutoFormatTable6"=37, "xlRangeAutoFormatTable7"=38, "xlRangeAutoFormatTable8"=39, "xlRangeAutoFormatTable9"=40, "xlRangeAutoFormatTable10"=41, "xlRangeAutoFormatPTNone"=42, "xlRangeAutoFormatNone"=-4142, "xlRangeAutoFormatSimple"=-4154] ("auto format (none)")
                                w833 = 1 items=["left", "center", "right"] ("horizontal alignment (left)")
                                w848 = 36 items=["xlRangeAutoFormat3DEffects1"=13, "xlRangeAutoFormat3DEffects2"=14, "xlRangeAutoFormatAccounting1"=4, "xlRangeAutoFormatAccounting2"=5, "xlRangeAutoFormatAccounting3"=6, "xlRangeAutoFormatAccounting4"=17, "xlRangeAutoFormatClassic1"=1, "xlRangeAutoFormatClassic2"=2, "xlRangeAutoFormatClassic3"=3, "xlRangeAutoFormatColor1"=7, "xlRangeAutoFormatColor2"=8, "xlRangeAutoFormatColor3"=9, "xlRangeAutoFormatList1"=10, "xlRangeAutoFormatList2"=11, "xlRangeAutoFormatList3"=12, "xlRangeAutoFormatLocalFormat1"=15, "xlRangeAutoFormatLocalFormat2"=16, "xlRangeAutoFormatLocalFormat3"=19, "xlRangeAutoFormatLocalFormat4"=20, "xlRangeAutoFormatReport1"=21, "xlRangeAutoFormatReport2"=22, "xlRangeAutoFormatReport3"=23, "xlRangeAutoFormatReport4"=24, "xlRangeAutoFormatReport5"=25, "xlRangeAutoFormatReport6"=26, "xlRangeAutoFormatReport7"=27, "xlRangeAutoFormatReport8"=28, "xlRangeAutoFormatReport9"=29, "xlRangeAutoFormatReport10"=30, "xlRangeAutoFormatClassicPivotTable"=31, "xlRangeAutoFormatTable1"=32, "xlRangeAutoFormatTable2"=33, "xlRangeAutoFormatTable3"=34, "xlRangeAutoFormatTable4"=35, "xlRangeAutoFormatTable5"=36, "xlRangeAutoFormatTable6"=37, "xlRangeAutoFormatTable7"=38, "xlRangeAutoFormatTable8"=39, "xlRangeAutoFormatTable9"=40, "xlRangeAutoFormatTable10"=41, "xlRangeAutoFormatPTNone"=42, "xlRangeAutoFormatNone"=-4142, "xlRangeAutoFormatSimple"=-4154] ("auto format (none)")
                                w842 = T25 3 items=["B&W", "4 bits", "8 bits", "24 bits"] ("image depth")
                                n525 = property on="Test Data table" class="Tbl (엄격한)"() -> ("Row Headers[]"=w850:string[])  [unwired: 2 in, 2 out]
                                n526 = local read "Test Data table"() -> (w838:string[][])
                                n527 = property on="Test Data table" class="Tbl (엄격한)"() -> ("Column Headers[]"=w849:string[])  [unwired: 2 in, 2 out]
                                n528 = Transpose 2D Array(2D array=w838) -> (transposed array=w847:string[][])
                                n529 = call <vilib>:"New Report.vi"("window state (normal)"=T20."normal", "report type"=T19."Excel") -> ("report out"=w845:refnum<class "NI_report.lvclass">, "error out"=w846:errorcluster)  [unwired: 12 in]
                                n530 = call-poly <vilib>:"Excel Easy Table.vi"("report in"=w845, "auto format (none)"=w848, "text data"=w847, "error in (no error)"=w846, "row headers"=w849, "column headers"=w850) -> ("report out"=w837:refnum<class "NI_report.lvclass">, "error out"=w836:errorcluster)  [unwired: 5 in, 3 out]
                                n531 = control-ref of="Load vs Ratio Graph"() -> (w841:refnum<vi>)
                                n532 = call <vilib>:"Excel Set Cell Alignment.vi"("report in"=w837, "horizontal alignment (left)"=w833, "error in (no error)"=w836) -> ("report out"=w835:refnum<class "NI_report.lvclass">, "error out"=w834:errorcluster)  [unwired: 11 in]
                                n533 = call-dynamic "Append Control Image to Report.vi"("report in"=w835, "image depth"=w842, "ctrl reference"=w841, "description"="Load vs Ratio Graph", "error in (no error)"=w834, "MS Office parameters"=T18 {"position (Excel)"={"row"=13, "column"=1}, "name (Excel)"="", "bookmark (Word)"=""}) -> ("report out"=w831:refnum<class "NI_report.lvclass">, "error out"=w830:errorcluster)  [unwired: 6 in, 2 out]
                                n534 = call-poly <vilib>:"Excel Easy Table.vi"("report in"=w831, "auto format (none)"=w829, "start (0, 0)"=cluster{"row":i32, "column":i32} {"row"=30, "column"=0}, "text data"=w825, "error in (no error)"=w830, "row headers"=w824, "column headers"=w823) -> ("report out"=w828:refnum<class "NI_report.lvclass">, "error out"=w827:errorcluster)  [unwired: 4 in, 3 out]
                                n535 = call-dynamic "Save Report to File.vi"("report in"=w828, "report file path"=w832, "error in (no error)"=w827) -> ()  [unwired: 11 in, 2 out]
                                }
                              }
                              n536 = control-ref of="Test Status"() -> (w764:refnum<vi>)
                              n537 = call "SUB-Status string update.vi"("텍스트 입력"="Result Data Process\n" ("Force Test Status"), "날짜추가"=TRUE, "reference"=w764) -> ()  [unwired: 2 in, 1 out]
                              n538 = local write "FTS OP status"(T6 "시험 종료" ("FTS 동작시험 상태")) -> ()
                            }
                            frame "시험 종료", Default {
                              # "시험 종료"
                              n539 = control-ref of="Test Status"() -> (w854:refnum<vi>)
                              n540 = local write "Mark10 Gauge (lb)"(0.0 ("Mark10 Gauge")) -> ()
                              n541 = local write "Clear graph 1"(TRUE ("그래프 지우기")) -> ()
                              n542 = call "SUB-Status string update.vi"("텍스트 입력"="Test complete." ("Force Test Status"), "날짜추가"=TRUE, "reference"=w854) -> ()  [unwired: 2 in, 1 out]
                              n543 = call <vilib>:"Beep.vi"() -> ()  [unwired: 12 in]
                            }
                          }
                        }
                      }
                      frame #3 {
                        n544 = local write "FTS comm."(FALSE ("FTS 수신 정상")) -> ()
                        n545 = local write "Test Start"(FALSE ("Test Start")) -> ()
                        n546 = local write "FTS Testing"(FALSE ("FTS 시험 진행")) -> ()
                      }
                    }
                  }
                }
              }
            }
          }
          frame #4 {
            # "설정값 읽기"
            n547 = disable-structure shown="비활성화" {
              frame Disabled {
                n548 = local read "Setting load(led)"() -> (w861:bool)
                n549 = local read "Comm con status 1"() -> (w860:bool)
                n550 = case shown="참" w861 {
                  tunnel: w860 -> [_ w862]
                  frame False {
                  }
                  frame True {
                    n551 = stacked-sequence {
                      tunnel: w862 -> [_ w864 _ _]
                      frame #0 {
                        n552 = local write "status string"("Loading setting values ..." ("status string")) -> ()
                      }
                      frame #1 {
                        n553 = case shown="참" w864 {
                          frame False {
                          }
                          frame True {
                            # "RS232"
                            n554 = stacked-sequence {
                              frame #0 {
                                n555 = local write "ACT-Comm"(TRUE ("ACT-RS422")) -> ()
                                n556 = local write "Data trx(led)"(TRUE ("Rx")) -> ()
                                n557 = local write "Rx-mon"(FALSE) -> ()
                              }
                              frame #1 {
                                n558 = call "SUB_Delay ms.vi"("delay(ms)"=u32 100 ("ms 배수")) -> ()  [unwired: 3 in]
                              }
                              frame #2 {
                                n559 = local read "Rx-mon"() -> (w871:bool)
                                n560 = case shown="참" w871 {
                                frame False {
                                }
                                frame True {
                                n561 = local write "Comm con status 1"(FALSE ("Connected")) -> ()
                                }
                                }
                                n562 = local write "ACT-Comm"(FALSE ("ACT-RS422")) -> ()
                                n563 = local write "Data trx(led)"(FALSE ("Rx")) -> ()
                              }
                            }
                          }
                        }
                      }
                      frame #2 {
                      }
                      frame #3 {
                        n564 = local write "Setting load(led)"(FALSE ("Power On Flag")) -> ()
                        n565 = local write "status string"("Complete call settings." ("status string")) -> ()
                        n566 = local write "Setting load"(FALSE ("Power On Flag")) -> ()
                      }
                    }
                  }
                }
              }
              frame Enabled {
              }
            }
          }
          frame #5 {
            # "설정값 저장"
            n567 = disable-structure shown="비활성화" {
              frame Disabled {
                n568 = local read "Comm con status 1"() -> (w876:bool)
                n569 = stacked-sequence {
                  tunnel: w876 -> [w877]
                  frame #0 {
                    n570 = case shown="참" w877 {
                      frame False {
                      }
                      frame True {
                        # "RS232"
                        n571 = stacked-sequence {
                          frame #0 {
                            n572 = disable-structure shown="비활성화" {
                              frame Disabled {
                                # "디지털 설정 Setpoint 레벨(0~100%)"
                                n573 = local read item#-1() -> (w879)
                                n574 = Equal?(x=w879, y=T21 "" ("설정값 선택")) -> (x = y?=w880:bool)
                                n575 = case shown="참" w880 {
                                frame False {
                                }
                                frame True {
                                n576 = local read item#-1() -> (w886)
                                n577 = local write "ACT-Comm"(TRUE ("ACT-RS422")) -> ()
                                n578 = Number To Fractional String(number=w886, precision (6)=i16 3 ("정밀도(6)")) -> (F-format string=w884:string)  [unwired: 2 in]
                                n579 = call <vilib>:"Space Constant.vi"() -> ("String"=w890:string)
                                n580 = local write "status string"("설정값 전송 - 디지털 설정 Setpoint" ("status string")) -> ()
                                n581 = local read "Port-act 1"() -> (w891:refnum<visa-resource-name>)
                                n582 = Concatenate Strings("SET_DIGSETPOINT" ("전송 문자열"), w890, w884) -> (w888:string)
                                n583 = call "_시리얼 데이타 전송.vi"("전송 문자열"=w888, "시리얼 포트"=w891) -> ()  [unwired: 2 out]
                                n584 = local write "Data trx(led)"(TRUE ("Rx")) -> ()
                                n585 = local write item#-1(T21 "" ("설정값 선택")) -> ()
                                }
                                }
                              }
                              frame Enabled {
                              }
                            }
                          }
                          frame #1 {
                            n586 = local read "ACT-Comm"() -> (w893:bool)
                            n587 = case shown="참" w893 {
                              frame False {
                              }
                              frame True {
                                n588 = flat-sequence {
                                frame #0 {
                                n589 = call "SUB_Delay ms.vi"("delay(ms)"=u32 100 ("ms 배수")) -> ()  [unwired: 3 in]
                                }
                                frame #1 {
                                n590 = local write "ACT-Comm"(FALSE ("ACT-RS422")) -> ()
                                }
                                }
                              }
                            }
                            n591 = local write "Data trx(led)"(FALSE ("Rx")) -> ()
                          }
                        }
                      }
                    }
                  }
                }
              }
              frame Enabled {
              }
            }
          }
          frame #6 {
            # "지연 시간, 상태값 리셋"
            n592 = local read "Comm con status 1"() -> (w901:bool)
            n593 = local read "Clear graph 1"() -> (w900:bool)
            n594 = Not(x=w901) -> (.not. x?=w898:bool)
            n595 = case shown="참" w898 {
              frame False {
              }
              frame True {
                n596 = local write "status string"("Ready (available after the communication connection)" ("status string")) -> ()
              }
            }
            n597 = case shown="참" w900 {
              frame False {
              }
              frame True {
                n598 = local write "Clear graph 1"(FALSE ("그래프 지우기")) -> ()
                n599 = property on="CDC(PCAP02) Graph" class="WFChart (엄격한)"("History Data"=waveform(dbl)[][] [] ("히스토리 데이터")) -> ()  [unwired: 2 in, 2 out]
              }
            }
            n600 = local read "Export graph 1"() -> (w899:bool)
            n601 = local read "Export graph2"() -> (w897:bool)
            n602 = local read "Clear graph 2"() -> (w896:bool)
            n603 = case shown="참" w897 {
              frame False {
              }
              frame True {
                n604 = invoke on="IMU Graph" class="WFChart (엄격한)" method="Export Data to Excel"() -> ()  [unwired: 3 in, 3 out]
                n605 = local write "Export graph2"(FALSE ("그래프 반출")) -> ()
              }
            }
            n606 = case shown="참" w899 {
              frame False {
              }
              frame True {
                n607 = invoke on="CDC(PCAP02) Graph" class="WFChart (엄격한)" method="Export Data to Excel"() -> ()  [unwired: 3 in, 3 out]
                n608 = local write "Export graph 1"(FALSE ("그래프 반출")) -> ()
              }
            }
            n609 = case shown="참" w896 {
              frame False {
              }
              frame True {
                n610 = local write "Clear graph 2"(FALSE ("그래프 지우기")) -> ()
                n611 = property on="IMU Graph" class="WFChart (엄격한)"("History Data"=waveform(dbl)[][] [] ("히스토리 데이터")) -> ()  [unwired: 2 in, 2 out]
              }
            }
          }
          frame #7 {
            # "옵셋 설정 (저장)"
            n612 = local read "Comm con status 1"() -> (w911:bool)
            n613 = local read "Comm con status 1"() -> (w912:bool)
            n614 = local read "Offset 2"() -> (w910:bool)
            n615 = local read "Offset 1"() -> (w913:bool)
            n616 = And(x=w911, y=w910) -> (x .and. y?=w909:bool)
            n617 = And(x=w912, y=w913) -> (x .and. y?=w914:bool)
            n618 = case shown="참" w909 {
              frame False {
                n619 = local write "Offset 2"(FALSE ("Offset 1")) -> ()
              }
              frame True {
                n620 = local write "Offset 2"(FALSE ("Offset 1")) -> ()
                n621 = local write "Clear graph 2"(TRUE ("그래프 지우기")) -> ()
                n622 = for {
                  N: 50 -> [_]
                  tunnel: [w972] -> w950 mode=indexing
                  tunnel: [w971] -> w951 mode=indexing
                  tunnel: [w970] -> w952 mode=indexing
                  tunnel: [w969] -> w953 mode=indexing
                  tunnel: [w968] -> w954 mode=indexing
                  tunnel: [w967] -> w955 mode=indexing
                  n623 = local read "IMU Offet"() -> (w966:T9)
                  n624 = call "SUB-BLE Rx Wait.vi"("Timeout(ms)"=u16 200) -> ("RxReady"=w973:bool)  [unwired: 4 in]
                  n625 = case shown="참" w973 {
                    tunnel: [w976 w977] -> w965
                    tunnel: w966 -> [w976 _]
                    frame False {
                    }
                    frame True {
                      n626 = call "SUB-BLE Rx data Classify.vi"() -> ("data out"=w978:u8[])  [unwired: 3 in, 2 out]
                      n627 = call "SUB-BLE Rx data-CDC IMU.vi"("data in"=w978) -> ("IMU data"=w977:T9)  [unwired: 4 in, 3 out]
                    }
                  }
                  n628 = Unbundle By Name(w965) -> ("Gyroscope X"=w972:dbl, "Gyroscope Y"=w971:dbl, "Gyroscope Z"=w970:dbl, "Accelerometer X"=w969:dbl, "Accelerometer Y"=w968:dbl, "Accelerometer Z"=w967:dbl)
                  n629 = Wait Until Next ms Multiple(millisecond multiple=u32 20 ("ms 배수")) -> ()  [unwired: 1 out]
                }
                n630 = call-poly <vilib>:"Mean.vi"("X"=w950) -> ("mean"=w957:dbl)  [unwired: 1 out]
                n631 = call-poly <vilib>:"Mean.vi"("X"=w951) -> ("mean"=w958:dbl)  [unwired: 1 out]
                n632 = call-poly <vilib>:"Mean.vi"("X"=w952) -> ("mean"=w959:dbl)  [unwired: 1 out]
                n633 = call-poly <vilib>:"Mean.vi"("X"=w953) -> ("mean"=w960:dbl)  [unwired: 1 out]
                n634 = call-poly <vilib>:"Mean.vi"("X"=w954) -> ("mean"=w961:dbl)  [unwired: 1 out]
                n635 = call-poly <vilib>:"Mean.vi"("X"=w955) -> ("mean"=w962:dbl)  [unwired: 1 out]
                n636 = Bundle By Name(cluster=T9 {"Gyroscope X"=0.0, "Gyroscope Y"=0.0, "Gyroscope Z"=0.0, "Accelerometer X"=0.0, "Accelerometer Y"=0.0, "Accelerometer Z"=0.0} ("IMU data"), "Gyroscope X"=w957, "Gyroscope Y"=w958, "Gyroscope Z"=w959, "Accelerometer X"=w960, "Accelerometer Y"=w961, "Accelerometer Z"=w962) -> (w956:T9)
                n637 = local write "IMU Offet"(w956) -> ()
              }
            }
            n638 = case shown="참" w914 {
              frame False {
                n639 = local write "Offset 1"(FALSE ("Offset 1")) -> ()
              }
              frame True {
                n640 = local write "Offset 1"(FALSE ("Offset 1")) -> ()
                n641 = local write "Clear graph 1"(TRUE ("그래프 지우기")) -> ()
                n642 = for {
                  N: 50 -> [_]
                  tunnel: [w940] -> w929 mode=indexing
                  tunnel: [w939] -> w928 mode=indexing
                  tunnel: [w938] -> w927 mode=indexing
                  tunnel: [w937] -> w926 mode=indexing
                  tunnel: [w936] -> w925 mode=indexing
                  tunnel: [w935] -> w924 mode=indexing
                  n643 = local read "CDC Offet"() -> (w933:T8)
                  n644 = call "SUB-BLE Rx Wait.vi"("Timeout(ms)"=u16 200) -> ("RxReady"=w941:bool)  [unwired: 4 in]
                  n645 = case shown="참" w941 {
                    tunnel: [w944 w945] -> w934
                    tunnel: w933 -> [w944 _]
                    frame False {
                    }
                    frame True {
                      n646 = call "SUB-BLE Rx data Classify.vi"() -> ("data out"=w946:u8[])  [unwired: 3 in, 2 out]
                      n647 = call "SUB-BLE Rx data-CDC IMU.vi"("data in"=w946) -> ("CDC data"=w945:T8)  [unwired: 4 in, 3 out]
                    }
                  }
                  n648 = Unbundle By Name(w934) -> ("Left Wing-A, C1/C0"=w940:dbl, "Left Wing-B, C2/C0"=w939:dbl, "Left Wing-C, C3/C0"=w938:dbl, "Right Wing-A, C4/C0"=w937:dbl, "Right Wing-B, C5/C0"=w936:dbl, "Right Wing-C, C6/C0"=w935:dbl)
                  n649 = Wait Until Next ms Multiple(millisecond multiple=u32 20 ("ms 배수")) -> ()  [unwired: 1 out]
                }
                n650 = call-poly <vilib>:"Mean.vi"("X"=w929) -> ("mean"=w921:dbl)  [unwired: 1 out]
                n651 = call-poly <vilib>:"Mean.vi"("X"=w928) -> ("mean"=w920:dbl)  [unwired: 1 out]
                n652 = call-poly <vilib>:"Mean.vi"("X"=w927) -> ("mean"=w919:dbl)  [unwired: 1 out]
                n653 = call-poly <vilib>:"Mean.vi"("X"=w926) -> ("mean"=w918:dbl)  [unwired: 1 out]
                n654 = call-poly <vilib>:"Mean.vi"("X"=w925) -> ("mean"=w917:dbl)  [unwired: 1 out]
                n655 = call-poly <vilib>:"Mean.vi"("X"=w924) -> ("mean"=w916:dbl)  [unwired: 1 out]
                n656 = Bundle By Name(cluster=T8 {"Left Wing-A, C1/C0"=0.0, "Left Wing-B, C2/C0"=0.0, "Left Wing-C, C3/C0"=0.0, "Right Wing-A, C4/C0"=0.0, "Right Wing-B, C5/C0"=0.0, "Right Wing-C, C6/C0"=0.0} ("CDC data"), "Left Wing-A, C1/C0"=w921, "Left Wing-B, C2/C0"=w920, "Left Wing-C, C3/C0"=w919, "Right Wing-A, C4/C0"=w918, "Right Wing-B, C5/C0"=w917, "Right Wing-C, C6/C0"=w916) -> (w922:T8)
                n657 = local write "CDC Offet"(w922) -> ()
              }
            }
          }
          frame #8 {
            # "데이터 로깅-GUI data"
            n658 = disable-structure shown="비활성화" {
              frame Disabled {
                n659 = local read "Data Logging"() -> (w979:bool)
                n660 = case shown="참" w979 {
                  frame False {
                    n661 = local read "Logging No."() -> (w981:u32)
                    n662 = Not Equal To 0?(x=w981) -> (x != 0?=w980:bool)
                    n663 = case shown="참" w980 {
                      frame False {
                      }
                      frame True {
                        n664 = local read "log refnum"() -> (w983:refnum<file>)
                        n665 = local write "Logging No."(u32 0 ("Logging No.")) -> ()
                        n666 = Close File(refnum=w983) -> ()  [unwired: 1 in, 2 out]
                      }
                    }
                  }
                  frame True {
                    n667 = stacked-sequence {
                      seq-local: [w984 _] -> [_ w1036]
                      frame #0 {
                        n668 = local read "IMU data"() -> (w987:T9)
                        n669 = local read "CDC data"() -> (w1004:T8)
                        n670 = Unbundle By Name(w1004) -> ("Left Wing-A, C1/C0"=w1001:dbl, "Left Wing-B, C2/C0"=w1000:dbl, "Left Wing-C, C3/C0"=w999:dbl, "Right Wing-A, C4/C0"=w998:dbl, "Right Wing-B, C5/C0"=w997:dbl, "Right Wing-C, C6/C0"=w996:dbl)
                        n671 = Unbundle By Name(w987) -> ("Gyroscope X"=w990:dbl, "Gyroscope Y"=w991:dbl, "Gyroscope Z"=w992:dbl, "Accelerometer X"=w993:dbl, "Accelerometer Y"=w994:dbl, "Accelerometer Z"=w995:dbl)
                        n672 = Format Into String(format string="%.7f,%.7f,%.7f,%.7f,%.7f,%.7f," ("포맷 문자열"), initial string=",,(GUI) CDC Data," ("포맷 문자열"), w1001, w1000, w999, w998, w997, w996) -> (resulting string=w986:string)  [unwired: 1 in, 1 out]
                        n673 = Format Into String(format string="%.6f,%.6f,%.6f,%.6f,%.6f,%.6f," ("포맷 문자열"), initial string=",(GUI) IMU Data," ("포맷 문자열"), w990, w991, w992, w993, w994, w995) -> (resulting string=w985:string)  [unwired: 1 in, 1 out]
                        n674 = Concatenate Strings(w986, w985) -> (w984:string)
                      }
                      frame #1 {
                        w1030 = T24 1 items=["사용자 홈"=0, "사용자 데스크탑"=1, "사용자 문서"=2, "사용자 어플리케이션 데이터"=3, "사용자 환경"=4, "사용자 임시"=5, "퍼블릭 문서"=6, "퍼블릭 어플리케이션 데이터"=7, "퍼블릭 환경"=8, "퍼블릭 캐시"=13, "시스템 코어 라이브러리"=9, "시스템 설치된 라이브러리"=10, "어플리케이션 파일"=11, "부팅 볼륨 루트"=12] ("system directory type")
                        # "첫행(타이틀)"
                        n675 = local read "Log no"() -> (w1005:string)
                        n676 = local read "Logging No."() -> (w1019:u32)
                        n677 = Format Date/Time String(time format string (%c)="Data Logging Start...  %Y/%m/%d %H:%M:%S" ("상태")) -> (date/time string=w1010:string)  [unwired: 2 in]
                        n678 = Format Into String(format string="\\\\GEN4 Data Logging(%s).csv" ("문자열"), w1005) -> (resulting string=w1006:string)  [unwired: 2 in, 1 out]
                        n679 = local read "RxD"() -> (w1040:string)
                        n680 = call <vilib>:"Get System Directory.vi"("system directory type"=w1030) -> ("system directory"=w1029:path)  [unwired: 10 in]
                        n681 = Format Into String(format string="\\r\\n\\r\\n%s\\r\\n%s\\r\\n" ("포맷 문자열"), w1010, "No.,Time,,Type,F/W ver.,(Raw)Left Wing-A,(Raw)Left Wing-B,(Raw)Left Wing-C,(Raw)Right Wing-A,(Raw)Right Wing-B,(Raw)Right Wing-C,(Raw)CDC Status,(Raw)Gyroscope X,(Raw)Gyroscope Y,(Raw)Gyroscope Z,(Raw)Accelerometer X,(Raw)Accelerometer Y,(Raw)Accelerometer Z,,Type,(GUI)Left Wing-A,(GUI)Left Wing-B,(GUI)Left Wing-C,(GUI)Right Wing-A,(GUI)Right Wing-B,(GUI)Right Wing-C,,Type,(GUI)Gyroscope X,(GUI)Gyroscope Y,(GUI)Gyroscope Z,(GUI)Accelerometer X,(GUI)Accelerometer Y,(GUI)Accelerometer Z" ("문자열")) -> (resulting string=w1008:string)  [unwired: 2 in, 1 out]
                        n682 = Increment(x=w1019) -> (x+1=w1035:u32)
                        n683 = Path To String(path=w1029) -> (string=w1028:string)
                        n684 = Equal To 0?(x=w1019) -> (x = 0?=w1017:bool)
                        n685 = Format Date/Time String(time format string (%c)="%Y/%m/%d %H:%M:%S%3u,,RXD Raw Data," ("상태")) -> (date/time string=w1042:string)  [unwired: 2 in]
                        n686 = Match Pattern(string=w1040, regular expression="#:" ("검색 문자열")) -> (after substring=w1038:string)  [unwired: 1 in, 3 out]
                        n687 = Format Into String(format string="%d," ("포맷 문자열"), w1019) -> (resulting string=w1033:string)  [unwired: 2 in, 1 out]
                        n688 = Concatenate Strings(w1028, w1006) -> (w1027:string)
                        n689 = local write "Logging No."(w1035) -> ()
                        n690 = String To Path(string=w1027) -> (path=w1026:path)
                        n691 = Open/Create/Replace File(file path (use dialog)=w1026, operation (0:open)=T22."open or create" ("동작(0:open)"), access (0:read/write)=enum16{"read/write", "read-only", "write-only"}."read/write" ("접근(0:읽기/쓰기)")) -> (refnum out=w1021:refnum<file>, error out=w1020:errorcluster)  [unwired: 3 in, 1 out]
                        n692 = Select(t=w1008, s=w1017, f="") -> (s? t:f=w1016:string)
                        n693 = Concatenate Strings(w1033, w1042, w1038, w1036, "\r\n") -> (w1015:string)
                        n694 = Get File Position(4:w1020, 7:w1021) -> (0:w1031:errorcluster, 2:w1018:i64, 3:w1032:refnum<file>)
                        n695 = Concatenate Strings(w1016, w1015) -> (w1014:string)
                        n696 = call <vilib>:"Write File+ (string).vi"("string"=w1014, "error in (no error)"=w1031, "pos offset (bytes:0)"=w1018, "refnum"=w1032) -> ("error out"=w1022:errorcluster, "dup refnum"=w1023:refnum<file>)  [unwired: 3 in, 1 out]
                        "log refnum" <- w1023
                        n697 = disable-structure shown="비활성화" {
                          disable-tunnel: w1023 -> [w1044 _]
                          disable-tunnel: w1022 -> [w1043 _]
                          frame Disabled {
                            n698 = Close File(refnum=w1044, error in=w1043) -> ()  [unwired: 2 out]
                          }
                          frame Enabled {
                          }
                        }
                      }
                    }
                  }
                }
              }
              frame Enabled {
              }
            }
          }
          frame #9 {
            # "데이터 로깅-BLE data"
            n699 = local read "Timer-ble log"() -> (w1051:u32)
            n700 = Tick Count (ms)() -> (millisecond timer value=w1052:u32)
            n701 = local read "log data1"() -> (w1049:bool)
            n702 = local read "Data Logging"() -> (w1050:bool)
            n703 = Subtract(x=w1052, y=w1051) -> (x-y=w1048:u32)
            n704 = Greater Or Equal?(x=w1048, y=u32 3000) -> (x >= y?=w1046:bool)
            n705 = Compound Arithmetic op=AND ("복합 연산")(w1050, w1049, w1046) -> (w1045:bool)
            n706 = case shown="참" w1045 {
              frame False {
              }
              frame True {
                n707 = stacked-sequence {
                  seq-local: [w1053 _ _] -> [_ _ w1058]
                  frame #0 {
                    n708 = local read "log ble buf"() -> (w1053:string)
                  }
                  frame #1 {
                    n709 = Tick Count (ms)() -> (millisecond timer value=w1056:u32)
                    n710 = local write "Timer-ble log"(w1056) -> ()
                    n711 = local write "log data1"(FALSE ("log data1")) -> ()
                    n712 = local write "log ble buf"("" ("log ble buf")) -> ()
                  }
                  frame #2 {
                    n713 = String Length(string=w1058) -> (length=w1057:i32)
                    n714 = case shown="1.." w1057 {
                      tunnel: w1058 -> [_ w1059]
                      frame 0, Default {
                      }
                      frame 1.. {
                        w1074 = T24 1 items=["사용자 홈"=0, "사용자 데스크탑"=1, "사용자 문서"=2, "사용자 어플리케이션 데이터"=3, "사용자 환경"=4, "사용자 임시"=5, "퍼블릭 문서"=6, "퍼블릭 어플리케이션 데이터"=7, "퍼블릭 환경"=8, "퍼블릭 캐시"=13, "시스템 코어 라이브러리"=9, "시스템 설치된 라이브러리"=10, "어플리케이션 파일"=11, "부팅 볼륨 루트"=12] ("system directory type")
                        n715 = local read "Log no"() -> (w1060:string)
                        n716 = Format Into String(format string="\\\\GEN4 BLE Data Logging(%s).txt" ("문자열"), w1060) -> (resulting string=w1061:string)  [unwired: 2 in, 1 out]
                        n717 = call <vilib>:"Get System Directory.vi"("system directory type"=w1074) -> ("system directory"=w1073:path)  [unwired: 10 in]
                        n718 = Path To String(path=w1073) -> (string=w1072:string)
                        n719 = Concatenate Strings(w1072, w1061) -> (w1071:string)
                        n720 = String To Path(string=w1071) -> (path=w1070:path)
                        n721 = Open/Create/Replace File(file path (use dialog)=w1070, operation (0:open)=T22."open or create" ("동작(0:open)"), access (0:read/write)=enum16{"read/write", "read-only", "write-only"}."read/write" ("접근(0:읽기/쓰기)")) -> (refnum out=w1065:refnum<file>, error out=w1064:errorcluster)  [unwired: 3 in, 1 out]
                        n722 = Get File Position(4:w1064, 7:w1065) -> (0:w1075:errorcluster, 2:w1063:i64, 3:w1076:refnum<file>)
                        n723 = call <vilib>:"Write File+ (string).vi"("string"=w1059, "error in (no error)"=w1075, "pos offset (bytes:0)"=w1063, "refnum"=w1076) -> ("error out"=w1066:errorcluster, "dup refnum"=w1067:refnum<file>)  [unwired: 3 in, 1 out]
                        n724 = disable-structure shown="비활성화" {
                          disable-tunnel: w1067 -> [w1078 _]
                          disable-tunnel: w1066 -> [w1077 _]
                          frame Disabled {
                            n725 = Close File(refnum=w1078, error in=w1077) -> ()  [unwired: 2 out]
                          }
                          frame Enabled {
                          }
                        }
                      }
                    }
                  }
                }
              }
            }
          }
          frame #10 {
            n726 = local write "Rx-mon"(FALSE) -> ()
          }
          frame #11 {
            # "디버깅 위해 창의 우측 크게 조정"
            # "창크게"
            n727 = local read "창크게"() -> (w1080:bool)
            n728 = case shown="참" w1080 {
              frame False {
              }
              frame True {
                n729 = First Call?() -> (First Call?: T/F=w1082:bool)
                n730 = case shown="참" w1082 {
                  frame False {
                  }
                  frame True {
                    w1099 = 250  # 확장 창 크기
                    n731 = Current VI's Path() -> (path=w1089:path)
                    n732 = Open VI Reference(vi path=w1089) -> (vi reference=w1090:refnum<vi>, error out=w1091:errorcluster)  [unwired: 5 in]
                    n733 = property class="VI"(reference=w1090, error in=w1091) -> (reference out=w1088:refnum<vi>, error out=w1086:errorcluster, "Front Panel.PanelBounds"=w1084:T26)
                    n734 = Unbundle By Name(w1084) -> ("Left"=w1098:i16, "Top"=w1096:i16, "Right"=w1094:i16, "Bottom"=w1095:i16)
                    n735 = expression code="x/2"(w1099) -> (w1093:i32)
                    n736 = Add(x=w1094, y=w1093) -> (x+y=w1092:i32)
                    n737 = Subtract(x=w1098, y=w1093) -> (x-y=w1097:i32)
                    n738 = Bundle By Name(cluster=w1084, "Left"=w1097, "Top"=w1096, "Right"=w1092, "Bottom"=w1095) -> (w1083:T26)
                    n739 = property class="VI"(reference=w1088, error in=w1086, "Front Panel.PanelBounds"=w1083) -> (reference out=w1087:refnum<vi>, error out=w1085:errorcluster)
                    n740 = Close Reference(reference=w1087, error in (no error)=w1085) -> ()  [unwired: 1 out]
                  }
                }
                n741 = local write "창크게"(FALSE ("창크게")) -> ()
              }
            }
          }
        }
        n742 = Wait Until Next ms Multiple(millisecond multiple=u32 4 ("ms 배수")) -> ()  [unwired: 1 out]
        n743 = local read "stop"() -> (w251:bool)
      }
      n744 = while {
        stop <- w227 stop-if-true
        # "값이 변경된 경우 데이타 전송 플레그=온"
        # "이벤트"
        n745 = event shown="[4] \"Data Logging\": 값 변경" {
          selector: _ -> [_ _ _ _ _ _]
          dyn-events: _ -> [_ _ _ _ _ _]
          timeout: 50 -> [_ _ _ _ _ _]
          event Timeout {
            n746 = event-data() -> ()  [unwired: 3 out]
          }
          event Key Down {
            # "Ctrl + 1"
            n747 = event-data() -> ("Char"=w235:i16, "VKey"=w233:T17, "Mods"=w237:cluster{"Num Pad":bool, "Menu Key":bool})  [unwired: 6 out]
            n748 = Unbundle By Name(w237) -> ("Menu Key"=w229:bool)
            n749 = Equal?(x=eventvkey."ASCII" ("V 키"), y=w233) -> (x = y?=w231:bool)
            n750 = Equal?(x=i16 49 ("문자"), y=w235) -> (x = y?=w232:bool)
            n751 = And(x=w232, y=w231) -> (x .and. y?=w230:bool)
            n752 = And(x=w230, y=w229) -> (x .and. y?=w228:bool)
            n753 = case shown="참" w228 {
              frame False {
              }
              frame True {
                n754 = local write "창크게"(TRUE ("창크게")) -> ()
              }
            }
          }
          event "Comm con 1": Value Change {
            n755 = event-data() -> ("NewVal"=w239:bool)  [unwired: 6 out]
            n756 = case shown="거짓" w239 {
              frame False {
                # "통신 닫기"
                n757 = local write "Port open 1"(FALSE) -> ()
                n758 = local write "Port close 1"(TRUE) -> ()
              }
              frame True {
                # "통신 연결"
                n759 = local write "Port open 1"(TRUE) -> ()
                n760 = local write "Port close 1"(FALSE) -> ()
              }
            }
          }
          event "Setting load": Value Change {
            n761 = event-data() -> ("NewVal"=w244:bool)  [unwired: 6 out]
            n762 = case shown="참" w244 {
              frame False {
              }
              frame True {
                n763 = local write "Setting load(led)"(TRUE ("Power On Flag")) -> ()
              }
            }
          }
          event "Data Logging": Value Change {
            n764 = event-data() -> ()  [unwired: 7 out]
            n765 = Tick Count (ms)() -> (millisecond timer value=w246:u32)
            n766 = local write "Timer-ble log"(w246) -> ()
          }
          event Panel Close? {
            n767 = event-data() -> ()  [unwired: 5 out]
            n768 = local write "stop"(TRUE ("stop")) -> ()
            n769 = event-data("Discard?"=TRUE ("stop")) -> ()  [unwired: 1 in, 1 out]
          }
        }
        n770 = local read "stop"() -> (w227:bool)
      }
      n771 = while {
        stop <- w148 stop-if-true
        # "BLE RxD handle"
        n772 = local read "Comm con status 1"() -> (w147:bool)
        n773 = local read "Port-act 1"() -> (w146:refnum<visa-resource-name>)
        n774 = case shown="참" w147 {
          tunnel: w146 -> [_ w153]
          frame False {
          }
          frame True {
            n775 = property class="Instr"(reference=w153) -> (reference out=w152:refnum<visa-resource-name>, error out=w151:errorcluster, "Serial Settings:Number of Bytes at Serial Port"=w150:u32)  [unwired: 1 in]
            n776 = case shown="4.." w150 {
              tunnel: w152 -> [_ w157]
              tunnel: w151 -> [_ w156]
              frame 0, Default {
                n777 = local write "Rx OK"(FALSE ("Rx OK")) -> ()
              }
              frame 4.. {
                # "Rx Packet Data - Process"
                n778 = call "ble_read_message.vi"("error in (no error)"=w156, "COM Bluegiga in"=w157) -> ("message package"=w155:u8[])  [unwired: 7 in, 2 out]
                n779 = stacked-sequence {
                  seq-local: [_ w161 _ _ _] -> [_ _ w184 w194 w199]
                  tunnel: w155 -> [_ w162 _ _ _]
                  frame #0 {
                    n780 = local write "Packet Detect"(FALSE ("Packet Detect")) -> ()
                  }
                  frame #1 {
                    # "ble_evt_attclient_attribute_value"
                    n781 = call "BLED1112-Rx Packet parser (EVENT-Attribute Client).vi"("message package"=w162) -> ("message out"=w161:u8[], "Packet OK"=w160:bool, "Data Structure"=w159:T1)  [unwired: 2 in]
                    n782 = case shown="참" w160 {
                      tunnel: w159 -> [_ w169]
                      frame False {
                      }
                      frame True {
                        n783 = local read "Data Logging"() -> (w165:bool)
                        n784 = Unbundle By Name(w169) -> ("Attribute value (data)"=w163:u8[])
                        n785 = Byte Array To String(unsigned byte array=w163) -> (string=w168:string)
                        n786 = call "SUB-BLE Rx data save.vi"("BLE RxD"=w163) -> ()  [unwired: 5 in]
                        n787 = local write "Rx buf 1"(w168) -> ()
                        n788 = local read "Rx Cnt"() -> (w164:i32)
                        n789 = case shown="참" w165 {
                          tunnel: w163 -> [_ w175]
                          tunnel: w164 -> [_ w172]
                          frame False {
                          }
                          frame True {
                            n790 = local read "log ble buf"() -> (w180:string)
                            n791 = Format Into String(format string="%06d  " ("포맷 문자열"), w172) -> (resulting string=w173:string)  [unwired: 2 in, 1 out]
                            n792 = call <vilib>:"Space Constant.vi"() -> ("String"=w171:string)
                            n793 = Array To Spreadsheet String(delimiter (Tab)=w171, array=w175, 3:"%02X" ("포맷 문자열")) -> (spreadsheet string=w176:string)
                            n794 = Format Date/Time String(time format string (%c)="%H:%M:%S%3u>  " ("상태")) -> (date/time string=w178:string)  [unwired: 2 in]
                            n795 = Concatenate Strings(w180, w173, w178, w176) -> (w179:string)
                            n796 = local write "log data1"(TRUE ("log data1")) -> ()
                            n797 = local write "log ble buf"(w179) -> ()
                          }
                        }
                        n798 = local write "Packet Detect"(TRUE ("Packet Detect")) -> ()
                        n799 = Increment(x=w164) -> (x+1=w170:i32)
                        n800 = local write "Rx Cnt"(w170) -> ()
                        n801 = local write "Rx OK"(TRUE ("Rx OK")) -> ()
                        "Rx Packet Structure" <- w169
                      }
                    }
                  }
                  frame #2 {
                    # "Rx Packet parser (EVENT-Connection status)"
                    n802 = local read "Packet Detect"() -> (w183:bool)
                    n803 = case shown="거짓" w183 {
                      tunnel: w184 -> [w187 _]
                      frame False {
                        n804 = call "BLED1112-Rx Packet parser (EVENT-Connection status).vi"("message package"=w187) -> ("Packet OK"=w186:bool, "Data Structure"=w185:T27)  [unwired: 2 in, 1 out]
                        n805 = case shown="참" w186 {
                          tunnel: w185 -> [_ w192]
                          frame False {
                          }
                          frame True {
                            n806 = Unbundle By Name(w192) -> ("bonding(0xFF)"=w191:u8)
                            n807 = local write "Packet Detect"(TRUE ("Packet Detect")) -> ()
                            n808 = Not Equal?(x=w191, y=255 ("Rx Cnt")) -> (x != y?=w189:bool)
                            n809 = local write "Disconnected"(w189) -> ()
                          }
                        }
                      }
                      frame True {
                      }
                    }
                  }
                  frame #3 {
                    # "Rx Packet parser (RESPONSE GAP)"
                    n810 = local read "Packet Detect"() -> (w193:bool)
                    n811 = case shown="거짓" w193 {
                      tunnel: w194 -> [w196 _]
                      frame False {
                        n812 = call "BLED1112-Rx Packet parser (RESPONSE-GAP).vi"("message package"=w196) -> ("Packet OK"=w195:bool)  [unwired: 2 in, 2 out]
                        n813 = case shown="참" w195 {
                          frame False {
                          }
                          frame True {
                            n814 = local write "Packet Detect"(TRUE ("Packet Detect")) -> ()
                          }
                        }
                      }
                      frame True {
                      }
                    }
                  }
                  frame #4 {
                    # "Rx Packet parser (EVENT-Disconnected)"
                    n815 = local read "Packet Detect"() -> (w198:bool)
                    n816 = case shown="거짓" w198 {
                      tunnel: w199 -> [w201 _]
                      frame False {
                        n817 = call "BLED1112-Rx Packet parser (EVENT-Disconnected).vi"("message package"=w201) -> ("Packet OK"=w202:bool, "Data Structure"=w200:T28)  [unwired: 2 in, 1 out]
                        n818 = case shown="참" w202 {
                          tunnel: w200 -> [_ _]
                          frame False {
                          }
                          frame True {
                            n819 = local write "Comm con status 1"(FALSE ("보드-통신상태 1")) -> ()
                            n820 = local write "Packet Detect"(TRUE ("Packet Detect")) -> ()
                            n821 = local write "Disconnected"(TRUE ("Disconnected")) -> ()
                            n822 = local write "ACT-Comm"(FALSE ("ACT-Comm")) -> ()
                            n823 = local write "Comm con 1"(FALSE ("보드 통신 연결 1")) -> ()
                            n824 = One Button Dialog(message="BLE Disconnected!" ("메시지")) -> ()  [unwired: 1 in, 1 out]
                          }
                        }
                      }
                      frame True {
                      }
                    }
                  }
                }
              }
            }
          }
        }
        n825 = Wait Until Next ms Multiple(millisecond multiple=u32 1 ("ms 배수")) -> ()  [unwired: 1 out]
        n826 = local read "stop"() -> (w148:bool)
      }
      n827 = while {
        stop <- w217 stop-if-true
        # "압력 시험"
        n828 = stacked-sequence {
          frame #0 {
            n829 = local read "Force Set"() -> (w219:bool)
            n830 = case shown="참" w219 {
              frame False {
              }
              frame True {
                n831 = stacked-sequence {
                  frame #0 {
                    n832 = local read "Port-FTS"() -> (w223:refnum<visa-resource-name>)
                    n833 = local read "Load(lb)"() -> (w222:dbl)
                    n834 = call "_시리얼_Mark10-제어 (압력설정).vi"("FTS 제어 상태"=T16 "압력제어 시작", "압력 설정(lb)"=w222, "시리얼 포트"=w223) -> ("통신 정상"=w220:bool)  [unwired: 2 out]
                    n835 = case shown="거짓" w220 {
                      frame False {
                        n836 = One Button Dialog(message="Can't find equipment!" ("메시지")) -> ()  [unwired: 1 in, 1 out]
                      }
                      frame True {
                      }
                    }
                  }
                  frame #1 {
                    n837 = local write "Force Set"(FALSE ("Force Set")) -> ()
                  }
                }
              }
            }
          }
        }
        n838 = Wait Until Next ms Multiple(millisecond multiple=u32 300 ("ms 배수")) -> ()  [unwired: 1 out]
        n839 = local read "stop"() -> (w217:bool)
      }
      n840 = while {
        stop <- w212 stop-if-true
        # "압력 시험-LED"
        n841 = local read "Force Set"() -> (w210:bool)
        n842 = local read "Test Start"() -> (w211:bool)
        n843 = Compound Arithmetic op=OR ("복합 연산")(w211, w210) -> (w209:bool)
        n844 = case shown="거짓" w209 {
          frame False {
            n845 = local write "FTS Testing"(FALSE ("FTS 시험 진행")) -> ()
          }
          frame True {
            n846 = local read "FTS Testing"() -> (w216:bool)
            n847 = Not(x=w216) -> (.not. x?=w215:bool)
            n848 = local write "FTS Testing"(w215) -> ()
          }
        }
        n849 = Wait Until Next ms Multiple(millisecond multiple=u32 300 ("ms 배수")) -> ()  [unwired: 1 out]
        n850 = local read "stop"() -> (w212:bool)
      }
    }
    frame #6 {
      # "시리얼 포트 닫기"
      n851 = local read "Comm con 1"() -> (w1100:bool)
      n852 = case shown="참" w1100 {
        frame False {
        }
        frame True {
          # "BLE 통신 종료"
          n853 = local read "Port-act 1"() -> (w1101:refnum<visa-resource-name>)
          n854 = local read "Connection Status"() -> (w1106:T4)
          n855 = call "_시리얼_buf clear.vi"("시리얼 포트"=w1101) -> ("에러 출력"=w1104:errorcluster, "시리얼 포트 2"=w1105:refnum<visa-resource-name>)  [unwired: 3 in]
          n856 = call "ble_disconnect_device.vi"("Connection Status"=w1106, "error in (no error)"=w1104, "COM Bluegiga in"=w1105) -> ("error out"=w1103:errorcluster, "COM Bluegiga out"=w1102:refnum<visa-resource-name>)  [unwired: 7 in]
          n857 = VISA Close(VISA resource name=w1102, error in (no error)=w1103) -> ()  [unwired: 1 out]
        }
      }
    }
    frame #7 {
      # "프로그램 설정값-파일로 저장한다."
      n858 = call <vilib>:"Open Config Data.vi"("configuration file path"=w1111) -> ("error out"=w1114:errorcluster, "refnum"=w1113:T23)  [unwired: 2 in, 7 out]
      n859 = stacked-sequence {
        tunnel: w1113 -> [w1118 w1121 w1126 w1131 w1136]
        tunnel: w1114 -> [w1117 w1120 w1125 w1130 w1135]
        tunnel: "GUI Setting" ("section") -> [w1119 w1122 w1127 w1132 _]
        tunnel: [_ _ _ _ w1136] -> w1110
        tunnel: [_ _ _ _ w1135] -> w1109
        frame #0 {
          w1116 = "Com Port-Board1"  # Key 1
          n860 = local read "Port-set 1"() -> (w1115:refnum<visa-resource-name>)
          n861 = call-poly <vilib>:"Write Key.vi"("section"=w1119, "error in (no error)"=w1117, "value"=w1115, "key"=w1116, "refnum"=w1118) -> ()  [unwired: 1 in, 6 out]
        }
        frame #1 {
          w1124 = "Com Port-FTS"  # Key 1
          n862 = local read "Port-FTS"() -> (w1123:refnum<visa-resource-name>)
          n863 = call-poly <vilib>:"Write Key.vi"("section"=w1122, "error in (no error)"=w1120, "value"=w1123, "key"=w1124, "refnum"=w1121) -> ()  [unwired: 1 in, 6 out]
        }
        frame #2 {
          w1129 = "Logno"  # Key 1
          n864 = local read "Log no"() -> (w1128:string)
          n865 = call-poly <vilib>:"Write Key.vi"("section"=w1127, "error in (no error)"=w1125, "value"=w1128, "key"=w1129, "refnum"=w1126) -> ()  [unwired: 1 in, 6 out]
        }
        frame #3 {
          w1134 = "Interval(ms)"  # Key 1
          n866 = local read "Interval(ms)"() -> (w1133:u16)
          n867 = call-poly <vilib>:"Write Key.vi"("section"=w1132, "error in (no error)"=w1130, "value"=w1133, "key"=w1134, "refnum"=w1131) -> ()  [unwired: 7 out]
        }
        frame #4 {
        }
      }
      n868 = call <vilib>:"Close Config Data.vi"("error in (no error)"=w1109, "refnum"=w1110) -> ()  [unwired: 1 in, 9 out]
      n869 = call "Read and Write Controls to Automatic Config File.vi"("Action"=RWC_Actions."Write", "Control References"=w1107) -> ()  [unwired: 9 in, 1 out]
    }
    frame #8 {
      # "종료"
      n870 = call "SUB-프런트패널 종료.vi"() -> ()  [unwired: 4 in]
    }
  }
  n871 = disable-structure shown="비활성화" {
    frame Disabled {
      n872 = local read "ms timer 2"() -> (w1139:u32)
      n873 = Tick Count (ms)() -> (millisecond timer value=w1140:u32)
      n874 = Concatenate Strings() -> (w1138:string, w1137:string)  [unwired: 1 in]
      n875 = Subtract(x=w1140, y=w1139) -> (x-y=w1141:u32)
      n876 = case shown="150.." w1141 {
        tunnel: w1138 -> [_ w1143]
        frame 0, Default {
        }
        frame 150.. {
          n877 = Tick Count (ms)() -> (millisecond timer value=w1142:u32)
          n878 = local write "RxD"(w1143) -> ()
          n879 = local write "ms timer 2"(w1142) -> ()
        }
      }
    }
    frame Enabled {
    }
  }
